vi "barcode main.vi"(8 "error in":errorcluster, 10 "bc station config":T1 {"LIN INFO"."NAD" format="%.0x"; "LIN INFO"."ADCS LIN"."HW select" items=["NI-XNET", "NI-CAN"]; "LVDT Status"."LVDT's stored config"."Lower Limit" format="%.2f"; "LVDT Status"."LVDT's stored config"."Upper Limit" format="%.2f"; "PLC Comms"."PLC string write Tags"."error message 9"."DataSocket Reference"."OnStatusUpdated" format="%.0x"; "PLC Comms"."PLC string write Tags"."error message 9"."DataSocket Reference"."OnDataUpdated" format="%.0x"; "PLC Comms"."PLC string write Tags"."error message 8"."DataSocket Reference"."OnStatusUpdated" format="%.0x"; "PLC Comms"."PLC string write Tags"."error message 8"."DataSocket Reference"."OnDataUpdated" format="%.0x"; "PLC Comms"."PLC string write Tags"."error message 7"."DataSocket Reference"."OnStatusUpdated" format="%.0x"; "PLC Comms"."PLC string write Tags"."error message 7"."DataSocket Reference"."OnDataUpdated" format="%.0x"; "PLC Comms"."PLC string write Tags"."error message 6"."DataSocket Reference"."OnStatusUpdated" format="%.0x"; "PLC Comms"."PLC string write Tags"."error message 6"."DataSocket Reference"."OnDataUpdated" format="%.0x"; "PLC Comms"."PLC string write Tags"."error message 5"."DataSocket Reference"."OnStatusUpdated" format="%.0x"; "PLC Comms"."PLC string write Tags"."error message 5"."DataSocket Reference"."OnDataUpdated" format="%.0x"; "PLC Comms"."PLC string write Tags"."error message 4"."DataSocket Reference"."OnStatusUpdated" format="%.0x"; "PLC Comms"."PLC string write Tags"."error message 4"."DataSocket Reference"."OnDataUpdated" format="%.0x"; "PLC Comms"."PLC string write Tags"."error message 3"."DataSocket Reference"."OnStatusUpdated" format="%.0x"; "PLC Comms"."PLC string write Tags"."error message 3"."DataSocket Reference"."OnDataUpdated" format="%.0x"; "PLC Comms"."PLC string write Tags"."error message 2"."DataSocket Reference"."OnStatusUpdated" format="%.0x"; "PLC Comms"."PLC string write Tags"."error message 2"."DataSocket Reference"."OnDataUpdated" format="%.0x"; "PLC Comms"."PLC string write Tags"."error message 1"."DataSocket Reference"."OnStatusUpdated" format="%.0x"; "PLC Comms"."PLC string write Tags"."error message 1"."DataSocket Reference"."OnDataUpdated" format="%.0x"; "PLC Comms"."PLC string write Tags"."error message 0"."DataSocket Reference"."OnStatusUpdated" format="%.0x"; "PLC Comms"."PLC string write Tags"."error message 0"."DataSocket Reference"."OnDataUpdated" format="%.0x"; "PLC Comms"."PLC string write Tags"."barcode station error"."DataSocket Reference"."OnStatusUpdated" format="%.0x"; "PLC Comms"."PLC string write Tags"."barcode station error"."DataSocket Reference"."OnDataUpdated" format="%.0x"; "PLC Comms"."PLC string read Tags"."iGPS SN 9"."DataSocket Reference"."OnStatusUpdated" format="%.0x"; "PLC Comms"."PLC string read Tags"."iGPS SN 9"."DataSocket Reference"."OnDataUpdated" format="%.0x"; "PLC Comms"."PLC string read Tags"."iGPS SN 8"."DataSocket Reference"."OnStatusUpdated" format="%.0x"; "PLC Comms"."PLC string read Tags"."iGPS SN 8"."DataSocket Reference"."OnDataUpdated" format="%.0x"; "PLC Comms"."PLC string read Tags"."iGPS SN 7"."DataSocket Reference"."OnStatusUpdated" format="%.0x"; "PLC Comms"."PLC string read Tags"."iGPS SN 7"."DataSocket Reference"."OnDataUpdated" format="%.0x"; "PLC Comms"."PLC string read Tags"."iGPS SN 6"."DataSocket Reference"."OnStatusUpdated" format="%.0x"; "PLC Comms"."PLC string read Tags"."iGPS SN 6"."DataSocket Reference"."OnDataUpdated" format="%.0x"; "PLC Comms"."PLC string read Tags"."iGPS SN 5"."DataSocket Reference"."OnStatusUpdated" format="%.0x"; "PLC Comms"."PLC string read Tags"."iGPS SN 5"."DataSocket Reference"."OnDataUpdated" format="%.0x"; "PLC Comms"."PLC string read Tags"."iGPS SN 4"."DataSocket Reference"."OnStatusUpdated" format="%.0x"; "PLC Comms"."PLC string read Tags"."iGPS SN 4"."DataSocket Reference"."OnDataUpdated" format="%.0x"; "PLC Comms"."PLC string read Tags"."iGPS SN 3"."DataSocket Reference"."OnStatusUpdated" format="%.0x"; "PLC Comms"."PLC string read Tags"."iGPS SN 3"."DataSocket Reference"."OnDataUpdated" format="%.0x"; "PLC Comms"."PLC string read Tags"."iGPS SN 2"."DataSocket Reference"."OnStatusUpdated" format="%.0x"; "PLC Comms"."PLC string read Tags"."iGPS SN 2"."DataSocket Reference"."OnDataUpdated" format="%.0x"; "PLC Comms"."PLC string read Tags"."iGPS SN 1"."DataSocket Reference"."OnStatusUpdated" format="%.0x"; "PLC Comms"."PLC string read Tags"."iGPS SN 1"."DataSocket Reference"."OnDataUpdated" format="%.0x"; "PLC Comms"."PLC string read Tags"."iGPS SN 0"."DataSocket Reference"."OnStatusUpdated" format="%.0x"; "PLC Comms"."PLC string read Tags"."iGPS SN 0"."DataSocket Reference"."OnDataUpdated" format="%.0x"; "PLC Comms"."PLC string read Tags"."Manual Part History Number"."DataSocket Reference"."OnStatusUpdated" format="%.0x"; "PLC Comms"."PLC string read Tags"."Manual Part History Number"."DataSocket Reference"."OnDataUpdated" format="%.0x"; "PLC Comms"."PLC string read Tags"."Manual Customer Number"."DataSocket Reference"."OnStatusUpdated" format="%.0x"; "PLC Comms"."PLC string read Tags"."Manual Customer Number"."DataSocket Reference"."OnDataUpdated" format="%.0x"; "PLC Comms"."PLC string read Tags"."Manual Model Type"."DataSocket Reference"."OnStatusUpdated" format="%.0x"; "PLC Comms"."PLC string read Tags"."Manual Model Type"."DataSocket Reference"."OnDataUpdated" format="%.0x"; "PLC Comms"."PLC string read Tags"."Manual Shade Color"."DataSocket Reference"."OnStatusUpdated" format="%.0x"; "PLC Comms"."PLC string read Tags"."Manual Shade Color"."DataSocket Reference"."OnDataUpdated" format="%.0x"; "PLC Comms"."PLC string read Tags"."Manual Inalfa Part Number"."DataSocket Reference"."OnStatusUpdated" format="%.0x"; "PLC Comms"."PLC string read Tags"."Manual Inalfa Part Number"."DataSocket Reference"."OnDataUpdated" format="%.0x"; "PLC Comms"."PLC string read Tags"."Manual Serial Number"."DataSocket Reference"."OnStatusUpdated" format="%.0x"; "PLC Comms"."PLC string read Tags"."Manual Serial Number"."DataSocket Reference"."OnDataUpdated" format="%.0x"; "PLC Comms"."PLC string read Tags"."Shade 2 Barcode"."DataSocket Reference"."OnStatusUpdated" format="%.0x"; "PLC Comms"."PLC string read Tags"."Shade 2 Barcode"."DataSocket Reference"."OnDataUpdated" format="%.0x"; "PLC Comms"."PLC string read Tags"."Shade 1 Barcode"."DataSocket Reference"."OnStatusUpdated" format="%.0x"; "PLC Comms"."PLC string read Tags"."Shade 1 Barcode"."DataSocket Reference"."OnDataUpdated" format="%.0x"; "PLC Comms"."PLC string read Tags"."Part History Number"."DataSocket Reference"."OnStatusUpdated" format="%.0x"; "PLC Comms"."PLC string read Tags"."Part History Number"."DataSocket Reference"."OnDataUpdated" format="%.0x"; "PLC Comms"."PLC string read Tags"."Customer Number"."DataSocket Reference"."OnStatusUpdated" format="%.0x"; "PLC Comms"."PLC string read Tags"."Customer Number"."DataSocket Reference"."OnDataUpdated" format="%.0x"; "PLC Comms"."PLC string read Tags"."Model Type"."DataSocket Reference"."OnStatusUpdated" format="%.0x"; "PLC Comms"."PLC string read Tags"."Model Type"."DataSocket Reference"."OnDataUpdated" format="%.0x"; "PLC Comms"."PLC string read Tags"."Shade Color"."DataSocket Reference"."OnStatusUpdated" format="%.0x"; "PLC Comms"."PLC string read Tags"."Shade Color"."DataSocket Reference"."OnDataUpdated" format="%.0x"; "PLC Comms"."PLC string read Tags"."Inalfa Part Number"."DataSocket Reference"."OnStatusUpdated" format="%.0x"; "PLC Comms"."PLC string read Tags"."Inalfa Part Number"."DataSocket Reference"."OnDataUpdated" format="%.0x"; "PLC Comms"."PLC string read Tags"."Pallet Number"."DataSocket Reference"."OnStatusUpdated" format="%.0x"; "PLC Comms"."PLC string read Tags"."Pallet Number"."DataSocket Reference"."OnDataUpdated" format="%.0x"; "PLC Comms"."PLC string read Tags"."Serial Number"."DataSocket Reference"."OnStatusUpdated" format="%.0x"; "PLC Comms"."PLC string read Tags"."Serial Number"."DataSocket Reference"."OnDataUpdated" format="%.0x"; "PLC Comms"."PLC bool write Tags"."Move LVDT Adjust Station"."DataSocket Reference"."OnStatusUpdated" format="%.0x"; "PLC Comms"."PLC bool write Tags"."Move LVDT Adjust Station"."DataSocket Reference"."OnDataUpdated" format="%.0x"; "PLC Comms"."PLC bool write Tags"."AT set to Vent ATS Home Pos"."DataSocket Reference"."OnStatusUpdated" format="%.0x"; "PLC Comms"."PLC bool write Tags"."AT set to Vent ATS Home Pos"."DataSocket Reference"."OnDataUpdated" format="%.0x"; "PLC Comms"."PLC bool write Tags"."AT set to Vent ATS Test Pos"."DataSocket Reference"."OnStatusUpdated" format="%.0x"; "PLC Comms"."PLC bool write Tags"."AT set to Vent ATS Test Pos"."DataSocket Reference"."OnDataUpdated" format="%.0x"; "PLC Comms"."PLC bool write Tags"."Barcode02 OK"."DataSocket Reference"."OnStatusUpdated" format="%.0x"; "PLC Comms"."PLC bool write Tags"."Barcode02 OK"."DataSocket Reference"."OnDataUpdated" format="%.0x"; "PLC Comms"."PLC bool write Tags"."Barcode01 OK"."DataSocket Reference"."OnStatusUpdated" format="%.0x"; "PLC Comms"."PLC bool write Tags"."Barcode01 OK"."DataSocket Reference"."OnDataUpdated" format="%.0x"; "PLC Comms"."PLC bool write Tags"."AT set wand 02 home pos"."DataSocket Reference"."OnStatusUpdated" format="%.0x"; "PLC Comms"."PLC bool write Tags"."AT set wand 02 home pos"."DataSocket Reference"."OnDataUpdated" format="%.0x"; "PLC Comms"."PLC bool write Tags"."AT set sunshade 02 wand up"."DataSocket Reference"."OnStatusUpdated" format="%.0x"; "PLC Comms"."PLC bool write Tags"."AT set sunshade 02 wand up"."DataSocket Reference"."OnDataUpdated" format="%.0x"; "PLC Comms"."PLC bool write Tags"."NVH Operator Finish"."DataSocket Reference"."OnStatusUpdated" format="%.0x"; "PLC Comms"."PLC bool write Tags"."NVH Operator Finish"."DataSocket Reference"."OnDataUpdated" format="%.0x"; "PLC Comms"."PLC bool write Tags"."NVH Operator Glass Close Noise"."DataSocket Reference"."OnStatusUpdated" format="%.0x"; "PLC Comms"."PLC bool write Tags"."NVH Operator Glass Close Noise"."DataSocket Reference"."OnDataUpdated" format="%.0x"; "PLC Comms"."PLC bool write Tags"."NVH Operator Glass Open Noise"."DataSocket Reference"."OnStatusUpdated" format="%.0x"; "PLC Comms"."PLC bool write Tags"."NVH Operator Glass Open Noise"."DataSocket Reference"."OnDataUpdated" format="%.0x"; "PLC Comms"."PLC bool write Tags"."NVH Operator Sunshade Close Noise"."DataSocket Reference"."OnStatusUpdated" format="%.0x"; "PLC Comms"."PLC bool write Tags"."NVH Operator Sunshade Close Noise"."DataSocket Reference"."OnDataUpdated" format="%.0x"; "PLC Comms"."PLC bool write Tags"."NVH Operator Sunshade Open Noise"."DataSocket Reference"."OnStatusUpdated" format="%.0x"; "PLC Comms"."PLC bool write Tags"."NVH Operator Sunshade Open Noise"."DataSocket Reference"."OnDataUpdated" format="%.0x"; "PLC Comms"."PLC bool write Tags"."NVH Operator Vent Close Noise"."DataSocket Reference"."OnStatusUpdated" format="%.0x"; "PLC Comms"."PLC bool write Tags"."NVH Operator Vent Close Noise"."DataSocket Reference"."OnDataUpdated" format="%.0x"; "PLC Comms"."PLC bool write Tags"."NVH Operator Vent Open Noise"."DataSocket Reference"."OnStatusUpdated" format="%.0x"; "PLC Comms"."PLC bool write Tags"."NVH Operator Vent Open Noise"."DataSocket Reference"."OnDataUpdated" format="%.0x"; "PLC Comms"."PLC bool write Tags"."NVH Operator Check"."DataSocket Reference"."OnStatusUpdated" format="%.0x"; "PLC Comms"."PLC bool write Tags"."NVH Operator Check"."DataSocket Reference"."OnDataUpdated" format="%.0x"; "PLC Comms"."PLC bool write Tags"."NVH Operator Fail"."DataSocket Reference"."OnStatusUpdated" format="%.0x"; "PLC Comms"."PLC bool write Tags"."NVH Operator Fail"."DataSocket Reference"."OnDataUpdated" format="%.0x"; "PLC Comms"."PLC bool write Tags"."NVH Operator Pass"."DataSocket Reference"."OnStatusUpdated" format="%.0x"; "PLC Comms"."PLC bool write Tags"."NVH Operator Pass"."DataSocket Reference"."OnDataUpdated" format="%.0x"; "PLC Comms"."PLC bool write Tags"."NVH Operator Express Rollo Opened02"."DataSocket Reference"."OnStatusUpdated" format="%.0x"; "PLC Comms"."PLC bool write Tags"."NVH Operator Express Rollo Opened02"."DataSocket Reference"."OnDataUpdated" format="%.0x"; "PLC Comms"."PLC bool write Tags"."NVH Operator Express Rollo Closed01"."DataSocket Reference"."OnStatusUpdated" format="%.0x"; "PLC Comms"."PLC bool write Tags"."NVH Operator Express Rollo Closed01"."DataSocket Reference"."OnDataUpdated" format="%.0x"; "PLC Comms"."PLC bool write Tags"."NVH Operator Express Rollo Opened01"."DataSocket Reference"."OnStatusUpdated" format="%.0x"; "PLC Comms"."PLC bool write Tags"."NVH Operator Express Rollo Opened01"."DataSocket Reference"."OnDataUpdated" format="%.0x"; "PLC Comms"."PLC bool write Tags"."NVH Operator Express Glass Closed"."DataSocket Reference"."OnStatusUpdated" format="%.0x"; "PLC Comms"."PLC bool write Tags"."NVH Operator Express Glass Closed"."DataSocket Reference"."OnDataUpdated" format="%.0x"; "PLC Comms"."PLC bool write Tags"."NVH Operator Express Glass Opened"."DataSocket Reference"."OnStatusUpdated" format="%.0x"; "PLC Comms"."PLC bool write Tags"."NVH Operator Express Glass Opened"."DataSocket Reference"."OnDataUpdated" format="%.0x"; "PLC Comms"."PLC bool write Tags"."NVH Fail"."DataSocket Reference"."OnStatusUpdated" format="%.0x"; "PLC Comms"."PLC bool write Tags"."NVH Fail"."DataSocket Reference"."OnDataUpdated" format="%.0x"; "PLC Comms"."PLC bool write Tags"."NVH Pass"."DataSocket Reference"."OnStatusUpdated" format="%.0x"; "PLC Comms"."PLC bool write Tags"."NVH Pass"."DataSocket Reference"."OnDataUpdated" format="%.0x"; "PLC Comms"."PLC bool write Tags"."NVH SunRoof Stop"."DataSocket Reference"."OnStatusUpdated" format="%.0x"; "PLC Comms"."PLC bool write Tags"."NVH SunRoof Stop"."DataSocket Reference"."OnDataUpdated" format="%.0x"; "PLC Comms"."PLC bool write Tags"."NVH SunRoof Moving"."DataSocket Reference"."OnStatusUpdated" format="%.0x"; "PLC Comms"."PLC bool write Tags"."NVH SunRoof Moving"."DataSocket Reference"."OnDataUpdated" format="%.0x"; "PLC Comms"."PLC bool write Tags"."Extend Z LVDTS"."DataSocket Reference"."OnStatusUpdated" format="%.0x"; "PLC Comms"."PLC bool write Tags"."Extend Z LVDTS"."DataSocket Reference"."OnDataUpdated" format="%.0x"; "PLC Comms"."PLC bool write Tags"."Bad Frame Barcode"."DataSocket Reference"."OnStatusUpdated" format="%.0x"; "PLC Comms"."PLC bool write Tags"."Bad Frame Barcode"."DataSocket Reference"."OnDataUpdated" format="%.0x"; "PLC Comms"."PLC bool write Tags"."Good Frame Barcode"."DataSocket Reference"."OnStatusUpdated" format="%.0x"; "PLC Comms"."PLC bool write Tags"."Good Frame Barcode"."DataSocket Reference"."OnDataUpdated" format="%.0x"; "PLC Comms"."PLC bool write Tags"."AT VentPMACExtended"."DataSocket Reference"."OnStatusUpdated" format="%.0x"; "PLC Comms"."PLC bool write Tags"."AT VentPMACExtended"."DataSocket Reference"."OnDataUpdated" format="%.0x"; "PLC Comms"."PLC bool write Tags"."AT VentPMACHome"."DataSocket Reference"."OnStatusUpdated" format="%.0x"; "PLC Comms"."PLC bool write Tags"."AT VentPMACHome"."DataSocket Reference"."OnDataUpdated" format="%.0x"; "PLC Comms"."PLC bool write Tags"."control slide stop"."DataSocket Reference"."OnStatusUpdated" format="%.0x"; "PLC Comms"."PLC bool write Tags"."control slide stop"."DataSocket Reference"."OnDataUpdated" format="%.0x"; "PLC Comms"."PLC bool write Tags"."control slide start"."DataSocket Reference"."OnStatusUpdated" format="%.0x"; "PLC Comms"."PLC bool write Tags"."control slide start"."DataSocket Reference"."OnDataUpdated" format="%.0x"; "PLC Comms"."PLC bool write Tags"."ss servo close"."DataSocket Reference"."OnStatusUpdated" format="%.0x"; "PLC Comms"."PLC bool write Tags"."ss servo close"."DataSocket Reference"."OnDataUpdated" format="%.0x"; "PLC Comms"."PLC bool write Tags"."ss servo open"."DataSocket Reference"."OnStatusUpdated" format="%.0x"; "PLC Comms"."PLC bool write Tags"."ss servo open"."DataSocket Reference"."OnDataUpdated" format="%.0x"; "PLC Comms"."PLC bool write Tags"."Extend LVDT's"."DataSocket Reference"."OnStatusUpdated" format="%.0x"; "PLC Comms"."PLC bool write Tags"."Extend LVDT's"."DataSocket Reference"."OnDataUpdated" format="%.0x"; "PLC Comms"."PLC bool write Tags"."Retract LVDT's"."DataSocket Reference"."OnStatusUpdated" format="%.0x"; "PLC Comms"."PLC bool write Tags"."Retract LVDT's"."DataSocket Reference"."OnDataUpdated" format="%.0x"; "PLC Comms"."PLC bool write Tags"."Test Started"."DataSocket Reference"."OnStatusUpdated" format="%.0x"; "PLC Comms"."PLC bool write Tags"."Test Started"."DataSocket Reference"."OnDataUpdated" format="%.0x"; "PLC Comms"."PLC bool write Tags"."Test Complete Fail"."DataSocket Reference"."OnStatusUpdated" format="%.0x"; "PLC Comms"."PLC bool write Tags"."Test Complete Fail"."DataSocket Reference"."OnDataUpdated" format="%.0x"; "PLC Comms"."PLC bool write Tags"."Test Complete Pass"."DataSocket Reference"."OnStatusUpdated" format="%.0x"; "PLC Comms"."PLC bool write Tags"."Test Complete Pass"."DataSocket Reference"."OnDataUpdated" format="%.0x"; "PLC Comms"."PLC bool write Tags"."AT set wand home pos"."DataSocket Reference"."OnStatusUpdated" format="%.0x"; "PLC Comms"."PLC bool write Tags"."AT set wand home pos"."DataSocket Reference"."OnDataUpdated" format="%.0x"; "PLC Comms"."PLC bool write Tags"."AT set sunshade wand lower"."DataSocket Reference"."OnStatusUpdated" format="%.0x"; "PLC Comms"."PLC bool write Tags"."AT set sunshade wand lower"."DataSocket Reference"."OnDataUpdated" format="%.0x"; "PLC Comms"."PLC bool write Tags"."AT set glass wand lower"."DataSocket Reference"."OnStatusUpdated" format="%.0x"; "PLC Comms"."PLC bool write Tags"."AT set glass wand lower"."DataSocket Reference"."OnDataUpdated" format="%.0x"; "PLC Comms"."PLC boolean read Tags"."Finish Adjust LVDT"."DataSocket Reference"."OnStatusUpdated" format="%.0x"; "PLC Comms"."PLC boolean read Tags"."Finish Adjust LVDT"."DataSocket Reference"."OnDataUpdated" format="%.0x"; "PLC Comms"."PLC boolean read Tags"."Start Adjust LVDT"."DataSocket Reference"."OnStatusUpdated" format="%.0x"; "PLC Comms"."PLC boolean read Tags"."Start Adjust LVDT"."DataSocket Reference"."OnDataUpdated" format="%.0x"; "PLC Comms"."PLC boolean read Tags"."AT at vent ATS Home pos"."DataSocket Reference"."OnStatusUpdated" format="%.0x"; "PLC Comms"."PLC boolean read Tags"."AT at vent ATS Home pos"."DataSocket Reference"."OnDataUpdated" format="%.0x"; "PLC Comms"."PLC boolean read Tags"."AT at vent ATS test pos"."DataSocket Reference"."OnStatusUpdated" format="%.0x"; "PLC Comms"."PLC boolean read Tags"."AT at vent ATS test pos"."DataSocket Reference"."OnDataUpdated" format="%.0x"; "PLC Comms"."PLC boolean read Tags"."NVH Operator Re-do"."DataSocket Reference"."OnStatusUpdated" format="%.0x"; "PLC Comms"."PLC boolean read Tags"."NVH Operator Re-do"."DataSocket Reference"."OnDataUpdated" format="%.0x"; "PLC Comms"."PLC boolean read Tags"."NVH Operator Express Glass Vent Close"."DataSocket Reference"."OnStatusUpdated" format="%.0x"; "PLC Comms"."PLC boolean read Tags"."NVH Operator Express Glass Vent Close"."DataSocket Reference"."OnDataUpdated" format="%.0x"; "PLC Comms"."PLC boolean read Tags"."NVH Operator Express Glass vent Open"."DataSocket Reference"."OnStatusUpdated" format="%.0x"; "PLC Comms"."PLC boolean read Tags"."NVH Operator Express Glass vent Open"."DataSocket Reference"."OnDataUpdated" format="%.0x"; "PLC Comms"."PLC boolean read Tags"."windproof position"."DataSocket Reference"."OnStatusUpdated" format="%.0x"; "PLC Comms"."PLC boolean read Tags"."windproof position"."DataSocket Reference"."OnDataUpdated" format="%.0x"; "PLC Comms"."PLC boolean read Tags"."AT in wand 02 home pos"."DataSocket Reference"."OnStatusUpdated" format="%.0x"; "PLC Comms"."PLC boolean read Tags"."AT in wand 02 home pos"."DataSocket Reference"."OnDataUpdated" format="%.0x"; "PLC Comms"."PLC boolean read Tags"."AT in sunshad 02 wand up pos"."DataSocket Reference"."OnStatusUpdated" format="%.0x"; "PLC Comms"."PLC boolean read Tags"."AT in sunshad 02 wand up pos"."DataSocket Reference"."OnDataUpdated" format="%.0x"; "PLC Comms"."PLC boolean read Tags"."AT shade 02 position"."DataSocket Reference"."OnStatusUpdated" format="%.0x"; "PLC Comms"."PLC boolean read Tags"."AT shade 02 position"."DataSocket Reference"."OnDataUpdated" format="%.0x"; "PLC Comms"."PLC boolean read Tags"."NVH Operator Check"."DataSocket Reference"."OnStatusUpdated" format="%.0x"; "PLC Comms"."PLC boolean read Tags"."NVH Operator Check"."DataSocket Reference"."OnDataUpdated" format="%.0x"; "PLC Comms"."PLC boolean read Tags"."NVH Operator Finish"."DataSocket Reference"."OnStatusUpdated" format="%.0x"; "PLC Comms"."PLC boolean read Tags"."NVH Operator Finish"."DataSocket Reference"."OnDataUpdated" format="%.0x"; "PLC Comms"."PLC boolean read Tags"."NVH Operator Glass Close Noise"."DataSocket Reference"."OnStatusUpdated" format="%.0x"; "PLC Comms"."PLC boolean read Tags"."NVH Operator Glass Close Noise"."DataSocket Reference"."OnDataUpdated" format="%.0x"; "PLC Comms"."PLC boolean read Tags"."NVH Operator Glass Open Noise"."DataSocket Reference"."OnStatusUpdated" format="%.0x"; "PLC Comms"."PLC boolean read Tags"."NVH Operator Glass Open Noise"."DataSocket Reference"."OnDataUpdated" format="%.0x"; "PLC Comms"."PLC boolean read Tags"."NVH Operator Sunshade Close Noise"."DataSocket Reference"."OnStatusUpdated" format="%.0x"; "PLC Comms"."PLC boolean read Tags"."NVH Operator Sunshade Close Noise"."DataSocket Reference"."OnDataUpdated" format="%.0x"; "PLC Comms"."PLC boolean read Tags"."NVH Operator Sunshade Open Noise"."DataSocket Reference"."OnStatusUpdated" format="%.0x"; "PLC Comms"."PLC boolean read Tags"."NVH Operator Sunshade Open Noise"."DataSocket Reference"."OnDataUpdated" format="%.0x"; "PLC Comms"."PLC boolean read Tags"."NVH Operator Vent Close Noise"."DataSocket Reference"."OnStatusUpdated" format="%.0x"; "PLC Comms"."PLC boolean read Tags"."NVH Operator Vent Close Noise"."DataSocket Reference"."OnDataUpdated" format="%.0x"; "PLC Comms"."PLC boolean read Tags"."NVH Operator Vent Open Noise"."DataSocket Reference"."OnStatusUpdated" format="%.0x"; "PLC Comms"."PLC boolean read Tags"."NVH Operator Vent Open Noise"."DataSocket Reference"."OnDataUpdated" format="%.0x"; "PLC Comms"."PLC boolean read Tags"."NVH Operator Express Rollo Close02"."DataSocket Reference"."OnStatusUpdated" format="%.0x"; "PLC Comms"."PLC boolean read Tags"."NVH Operator Express Rollo Close02"."DataSocket Reference"."OnDataUpdated" format="%.0x"; "PLC Comms"."PLC boolean read Tags"."NVH Operator Express Rollo Open02"."DataSocket Reference"."OnStatusUpdated" format="%.0x"; "PLC Comms"."PLC boolean read Tags"."NVH Operator Express Rollo Open02"."DataSocket Reference"."OnDataUpdated" format="%.0x"; "PLC Comms"."PLC boolean read Tags"."NVH Operator Express Rollo Close01"."DataSocket Reference"."OnStatusUpdated" format="%.0x"; "PLC Comms"."PLC boolean read Tags"."NVH Operator Express Rollo Close01"."DataSocket Reference"."OnDataUpdated" format="%.0x"; "PLC Comms"."PLC boolean read Tags"."NVH Operator Express Rollo Open01"."DataSocket Reference"."OnStatusUpdated" format="%.0x"; "PLC Comms"."PLC boolean read Tags"."NVH Operator Express Rollo Open01"."DataSocket Reference"."OnDataUpdated" format="%.0x"; "PLC Comms"."PLC boolean read Tags"."NVH Operator Express Glass Close"."DataSocket Reference"."OnStatusUpdated" format="%.0x"; "PLC Comms"."PLC boolean read Tags"."NVH Operator Express Glass Close"."DataSocket Reference"."OnDataUpdated" format="%.0x"; "PLC Comms"."PLC boolean read Tags"."NVH Operator Express Glass Open"."DataSocket Reference"."OnStatusUpdated" format="%.0x"; "PLC Comms"."PLC boolean read Tags"."NVH Operator Express Glass Open"."DataSocket Reference"."OnDataUpdated" format="%.0x"; "PLC Comms"."PLC boolean read Tags"."NVH Operator Fail"."DataSocket Reference"."OnStatusUpdated" format="%.0x"; "PLC Comms"."PLC boolean read Tags"."NVH Operator Fail"."DataSocket Reference"."OnDataUpdated" format="%.0x"; "PLC Comms"."PLC boolean read Tags"."NVH Operator Pass"."DataSocket Reference"."OnStatusUpdated" format="%.0x"; "PLC Comms"."PLC boolean read Tags"."NVH Operator Pass"."DataSocket Reference"."OnDataUpdated" format="%.0x"; "PLC Comms"."PLC boolean read Tags"."Z LVDTs Extended"."DataSocket Reference"."OnStatusUpdated" format="%.0x"; "PLC Comms"."PLC boolean read Tags"."Z LVDTs Extended"."DataSocket Reference"."OnDataUpdated" format="%.0x"; "PLC Comms"."PLC boolean read Tags"."iGPS Pass 9"."DataSocket Reference"."OnStatusUpdated" format="%.0x"; "PLC Comms"."PLC boolean read Tags"."iGPS Pass 9"."DataSocket Reference"."OnDataUpdated" format="%.0x"; "PLC Comms"."PLC boolean read Tags"."iGPS Pass 8"."DataSocket Reference"."OnStatusUpdated" format="%.0x"; "PLC Comms"."PLC boolean read Tags"."iGPS Pass 8"."DataSocket Reference"."OnDataUpdated" format="%.0x"; "PLC Comms"."PLC boolean read Tags"."iGPS Pass 7"."DataSocket Reference"."OnStatusUpdated" format="%.0x"; "PLC Comms"."PLC boolean read Tags"."iGPS Pass 7"."DataSocket Reference"."OnDataUpdated" format="%.0x"; "PLC Comms"."PLC boolean read Tags"."iGPS Pass 6"."DataSocket Reference"."OnStatusUpdated" format="%.0x"; "PLC Comms"."PLC boolean read Tags"."iGPS Pass 6"."DataSocket Reference"."OnDataUpdated" format="%.0x"; "PLC Comms"."PLC boolean read Tags"."iGPS Pass 5"."DataSocket Reference"."OnStatusUpdated" format="%.0x"; "PLC Comms"."PLC boolean read Tags"."iGPS Pass 5"."DataSocket Reference"."OnDataUpdated" format="%.0x"; "PLC Comms"."PLC boolean read Tags"."iGPS Pass 4"."DataSocket Reference"."OnStatusUpdated" format="%.0x"; "PLC Comms"."PLC boolean read Tags"."iGPS Pass 4"."DataSocket Reference"."OnDataUpdated" format="%.0x"; "PLC Comms"."PLC boolean read Tags"."iGPS Pass 3"."DataSocket Reference"."OnStatusUpdated" format="%.0x"; "PLC Comms"."PLC boolean read Tags"."iGPS Pass 3"."DataSocket Reference"."OnDataUpdated" format="%.0x"; "PLC Comms"."PLC boolean read Tags"."iGPS Pass 2"."DataSocket Reference"."OnStatusUpdated" format="%.0x"; "PLC Comms"."PLC boolean read Tags"."iGPS Pass 2"."DataSocket Reference"."OnDataUpdated" format="%.0x"; "PLC Comms"."PLC boolean read Tags"."iGPS Pass 1"."DataSocket Reference"."OnStatusUpdated" format="%.0x"; "PLC Comms"."PLC boolean read Tags"."iGPS Pass 1"."DataSocket Reference"."OnDataUpdated" format="%.0x"; "PLC Comms"."PLC boolean read Tags"."iGPS Pass 0"."DataSocket Reference"."OnStatusUpdated" format="%.0x"; "PLC Comms"."PLC boolean read Tags"."iGPS Pass 0"."DataSocket Reference"."OnDataUpdated" format="%.0x"; "PLC Comms"."PLC boolean read Tags"."Check Frame Barcode"."DataSocket Reference"."OnStatusUpdated" format="%.0x"; "PLC Comms"."PLC boolean read Tags"."Check Frame Barcode"."DataSocket Reference"."OnDataUpdated" format="%.0x"; "PLC Comms"."PLC boolean read Tags"."SS Barcode Scanner Bypassed"."DataSocket Reference"."OnStatusUpdated" format="%.0x"; "PLC Comms"."PLC boolean read Tags"."SS Barcode Scanner Bypassed"."DataSocket Reference"."OnDataUpdated" format="%.0x"; "PLC Comms"."PLC boolean read Tags"."AT VentPMACisExtend"."DataSocket Reference"."OnStatusUpdated" format="%.0x"; "PLC Comms"."PLC boolean read Tags"."AT VentPMACisExtend"."DataSocket Reference"."OnDataUpdated" format="%.0x"; "PLC Comms"."PLC boolean read Tags"."AT VentPMACatHome"."DataSocket Reference"."OnStatusUpdated" format="%.0x"; "PLC Comms"."PLC boolean read Tags"."AT VentPMACatHome"."DataSocket Reference"."OnDataUpdated" format="%.0x"; "PLC Comms"."PLC boolean read Tags"."wind deflector low speed pos"."DataSocket Reference"."OnStatusUpdated" format="%.0x"; "PLC Comms"."PLC boolean read Tags"."wind deflector low speed pos"."DataSocket Reference"."OnDataUpdated" format="%.0x"; "PLC Comms"."PLC boolean read Tags"."wind deflector high speed pos"."DataSocket Reference"."OnStatusUpdated" format="%.0x"; "PLC Comms"."PLC boolean read Tags"."wind deflector high speed pos"."DataSocket Reference"."OnDataUpdated" format="%.0x"; "PLC Comms"."PLC boolean read Tags"."control slide right over stroke"."DataSocket Reference"."OnStatusUpdated" format="%.0x"; "PLC Comms"."PLC boolean read Tags"."control slide right over stroke"."DataSocket Reference"."OnDataUpdated" format="%.0x"; "PLC Comms"."PLC boolean read Tags"."control slide right good"."DataSocket Reference"."OnStatusUpdated" format="%.0x"; "PLC Comms"."PLC boolean read Tags"."control slide right good"."DataSocket Reference"."OnDataUpdated" format="%.0x"; "PLC Comms"."PLC boolean read Tags"."control slide left over stroke"."DataSocket Reference"."OnStatusUpdated" format="%.0x"; "PLC Comms"."PLC boolean read Tags"."control slide left over stroke"."DataSocket Reference"."OnDataUpdated" format="%.0x"; "PLC Comms"."PLC boolean read Tags"."control slide left good"."DataSocket Reference"."OnStatusUpdated" format="%.0x"; "PLC Comms"."PLC boolean read Tags"."control slide left good"."DataSocket Reference"."OnDataUpdated" format="%.0x"; "PLC Comms"."PLC boolean read Tags"."control slide at home"."DataSocket Reference"."OnStatusUpdated" format="%.0x"; "PLC Comms"."PLC boolean read Tags"."control slide at home"."DataSocket Reference"."OnDataUpdated" format="%.0x"; "PLC Comms"."PLC boolean read Tags"."ss servo closing"."DataSocket Reference"."OnStatusUpdated" format="%.0x"; "PLC Comms"."PLC boolean read Tags"."ss servo closing"."DataSocket Reference"."OnDataUpdated" format="%.0x"; "PLC Comms"."PLC boolean read Tags"."ss servo opening"."DataSocket Reference"."OnStatusUpdated" format="%.0x"; "PLC Comms"."PLC boolean read Tags"."ss servo opening"."DataSocket Reference"."OnDataUpdated" format="%.0x"; "PLC Comms"."PLC boolean read Tags"."ss servo at close"."DataSocket Reference"."OnStatusUpdated" format="%.0x"; "PLC Comms"."PLC boolean read Tags"."ss servo at close"."DataSocket Reference"."OnDataUpdated" format="%.0x"; "PLC Comms"."PLC boolean read Tags"."ss servo at open"."DataSocket Reference"."OnStatusUpdated" format="%.0x"; "PLC Comms"."PLC boolean read Tags"."ss servo at open"."DataSocket Reference"."OnDataUpdated" format="%.0x"; "PLC Comms"."PLC boolean read Tags"."manual barcode print"."DataSocket Reference"."OnStatusUpdated" format="%.0x"; "PLC Comms"."PLC boolean read Tags"."manual barcode print"."DataSocket Reference"."OnDataUpdated" format="%.0x"; "PLC Comms"."PLC boolean read Tags"."LVDT's Retracted"."DataSocket Reference"."OnStatusUpdated" format="%.0x"; "PLC Comms"."PLC boolean read Tags"."LVDT's Retracted"."DataSocket Reference"."OnDataUpdated" format="%.0x"; "PLC Comms"."PLC boolean read Tags"."abort"."DataSocket Reference"."OnStatusUpdated" format="%.0x"; "PLC Comms"."PLC boolean read Tags"."abort"."DataSocket Reference"."OnDataUpdated" format="%.0x"; "PLC Comms"."PLC boolean read Tags"."start"."DataSocket Reference"."OnStatusUpdated" format="%.0x"; "PLC Comms"."PLC boolean read Tags"."start"."DataSocket Reference"."OnDataUpdated" format="%.0x"; "PLC Comms"."PLC boolean read Tags"."bolt check 21"."DataSocket Reference"."OnStatusUpdated" format="%.0x"; "PLC Comms"."PLC boolean read Tags"."bolt check 21"."DataSocket Reference"."OnDataUpdated" format="%.0x"; "PLC Comms"."PLC boolean read Tags"."bolt check 20"."DataSocket Reference"."OnStatusUpdated" format="%.0x"; "PLC Comms"."PLC boolean read Tags"."bolt check 20"."DataSocket Reference"."OnDataUpdated" format="%.0x"; "PLC Comms"."PLC boolean read Tags"."bolt check 19"."DataSocket Reference"."OnStatusUpdated" format="%.0x"; "PLC Comms"."PLC boolean read Tags"."bolt check 19"."DataSocket Reference"."OnDataUpdated" format="%.0x"; "PLC Comms"."PLC boolean read Tags"."bolt check 18"."DataSocket Reference"."OnStatusUpdated" format="%.0x"; "PLC Comms"."PLC boolean read Tags"."bolt check 18"."DataSocket Reference"."OnDataUpdated" format="%.0x"; "PLC Comms"."PLC boolean read Tags"."bolt check 17"."DataSocket Reference"."OnStatusUpdated" format="%.0x"; "PLC Comms"."PLC boolean read Tags"."bolt check 17"."DataSocket Reference"."OnDataUpdated" format="%.0x"; "PLC Comms"."PLC boolean read Tags"."bolt check 16"."DataSocket Reference"."OnStatusUpdated" format="%.0x"; "PLC Comms"."PLC boolean read Tags"."bolt check 16"."DataSocket Reference"."OnDataUpdated" format="%.0x"; "PLC Comms"."PLC boolean read Tags"."bolt check 15"."DataSocket Reference"."OnStatusUpdated" format="%.0x"; "PLC Comms"."PLC boolean read Tags"."bolt check 15"."DataSocket Reference"."OnDataUpdated" format="%.0x"; "PLC Comms"."PLC boolean read Tags"."bolt check 14"."DataSocket Reference"."OnStatusUpdated" format="%.0x"; "PLC Comms"."PLC boolean read Tags"."bolt check 14"."DataSocket Reference"."OnDataUpdated" format="%.0x"; "PLC Comms"."PLC boolean read Tags"."bolt check 13"."DataSocket Reference"."OnStatusUpdated" format="%.0x"; "PLC Comms"."PLC boolean read Tags"."bolt check 13"."DataSocket Reference"."OnDataUpdated" format="%.0x"; "PLC Comms"."PLC boolean read Tags"."bolt check 12"."DataSocket Reference"."OnStatusUpdated" format="%.0x"; "PLC Comms"."PLC boolean read Tags"."bolt check 12"."DataSocket Reference"."OnDataUpdated" format="%.0x"; "PLC Comms"."PLC boolean read Tags"."bolt check 11"."DataSocket Reference"."OnStatusUpdated" format="%.0x"; "PLC Comms"."PLC boolean read Tags"."bolt check 11"."DataSocket Reference"."OnDataUpdated" format="%.0x"; "PLC Comms"."PLC boolean read Tags"."bolt check 10"."DataSocket Reference"."OnStatusUpdated" format="%.0x"; "PLC Comms"."PLC boolean read Tags"."bolt check 10"."DataSocket Reference"."OnDataUpdated" format="%.0x"; "PLC Comms"."PLC boolean read Tags"."bolt check 9"."DataSocket Reference"."OnStatusUpdated" format="%.0x"; "PLC Comms"."PLC boolean read Tags"."bolt check 9"."DataSocket Reference"."OnDataUpdated" format="%.0x"; "PLC Comms"."PLC boolean read Tags"."bolt check 8"."DataSocket Reference"."OnStatusUpdated" format="%.0x"; "PLC Comms"."PLC boolean read Tags"."bolt check 8"."DataSocket Reference"."OnDataUpdated" format="%.0x"; "PLC Comms"."PLC boolean read Tags"."bolt check 7"."DataSocket Reference"."OnStatusUpdated" format="%.0x"; "PLC Comms"."PLC boolean read Tags"."bolt check 7"."DataSocket Reference"."OnDataUpdated" format="%.0x"; "PLC Comms"."PLC boolean read Tags"."bolt check 6"."DataSocket Reference"."OnStatusUpdated" format="%.0x"; "PLC Comms"."PLC boolean read Tags"."bolt check 6"."DataSocket Reference"."OnDataUpdated" format="%.0x"; "PLC Comms"."PLC boolean read Tags"."bolt check 5"."DataSocket Reference"."OnStatusUpdated" format="%.0x"; "PLC Comms"."PLC boolean read Tags"."bolt check 5"."DataSocket Reference"."OnDataUpdated" format="%.0x"; "PLC Comms"."PLC boolean read Tags"."bolt check 4"."DataSocket Reference"."OnStatusUpdated" format="%.0x"; "PLC Comms"."PLC boolean read Tags"."bolt check 4"."DataSocket Reference"."OnDataUpdated" format="%.0x"; "PLC Comms"."PLC boolean read Tags"."bolt check 3"."DataSocket Reference"."OnStatusUpdated" format="%.0x"; "PLC Comms"."PLC boolean read Tags"."bolt check 3"."DataSocket Reference"."OnDataUpdated" format="%.0x"; "PLC Comms"."PLC boolean read Tags"."bolt check 2"."DataSocket Reference"."OnStatusUpdated" format="%.0x"; "PLC Comms"."PLC boolean read Tags"."bolt check 2"."DataSocket Reference"."OnDataUpdated" format="%.0x"; "PLC Comms"."PLC boolean read Tags"."bolt check 1"."DataSocket Reference"."OnStatusUpdated" format="%.0x"; "PLC Comms"."PLC boolean read Tags"."bolt check 1"."DataSocket Reference"."OnDataUpdated" format="%.0x"; "PLC Comms"."PLC boolean read Tags"."FB light block present"."DataSocket Reference"."OnStatusUpdated" format="%.0x"; "PLC Comms"."PLC boolean read Tags"."FB light block present"."DataSocket Reference"."OnDataUpdated" format="%.0x"; "PLC Comms"."PLC boolean read Tags"."audit gap hider present RH"."DataSocket Reference"."OnStatusUpdated" format="%.0x"; "PLC Comms"."PLC boolean read Tags"."audit gap hider present RH"."DataSocket Reference"."OnDataUpdated" format="%.0x"; "PLC Comms"."PLC boolean read Tags"."audit gap hider present LH"."DataSocket Reference"."OnStatusUpdated" format="%.0x"; "PLC Comms"."PLC boolean read Tags"."audit gap hider present LH"."DataSocket Reference"."OnDataUpdated" format="%.0x"; "PLC Comms"."PLC boolean read Tags"."motor foam present RH"."DataSocket Reference"."OnStatusUpdated" format="%.0x"; "PLC Comms"."PLC boolean read Tags"."motor foam present RH"."DataSocket Reference"."OnDataUpdated" format="%.0x"; "PLC Comms"."PLC boolean read Tags"."motor foam present LH"."DataSocket Reference"."OnStatusUpdated" format="%.0x"; "PLC Comms"."PLC boolean read Tags"."motor foam present LH"."DataSocket Reference"."OnDataUpdated" format="%.0x"; "PLC Comms"."PLC boolean read Tags"."LVDT's Extended"."DataSocket Reference"."OnStatusUpdated" format="%.0x"; "PLC Comms"."PLC boolean read Tags"."LVDT's Extended"."DataSocket Reference"."OnDataUpdated" format="%.0x"; "PLC Comms"."PLC boolean read Tags"."AT in wand home pos"."DataSocket Reference"."OnStatusUpdated" format="%.0x"; "PLC Comms"."PLC boolean read Tags"."AT in wand home pos"."DataSocket Reference"."OnDataUpdated" format="%.0x"; "PLC Comms"."PLC boolean read Tags"."AT in sunshad wand lower pos"."DataSocket Reference"."OnStatusUpdated" format="%.0x"; "PLC Comms"."PLC boolean read Tags"."AT in sunshad wand lower pos"."DataSocket Reference"."OnDataUpdated" format="%.0x"; "PLC Comms"."PLC boolean read Tags"."AT in glass wand lower pos"."DataSocket Reference"."OnStatusUpdated" format="%.0x"; "PLC Comms"."PLC boolean read Tags"."AT in glass wand lower pos"."DataSocket Reference"."OnDataUpdated" format="%.0x"; "PLC Comms"."PLC boolean read Tags"."AT shade position"."DataSocket Reference"."OnStatusUpdated" format="%.0x"; "PLC Comms"."PLC boolean read Tags"."AT shade position"."DataSocket Reference"."OnDataUpdated" format="%.0x"; "PLC Comms"."PLC boolean read Tags"."AT glass position"."DataSocket Reference"."OnStatusUpdated" format="%.0x"; "PLC Comms"."PLC boolean read Tags"."AT glass position"."DataSocket Reference"."OnDataUpdated" format="%.0x"; "Store Data"."Sun Shade Open Force Limits"."Variance" format="%.2g"; "Store Data"."Sun Shade Open Force Limits"."Truncation End" format="%.2g"; "Store Data"."Sun Shade Open Force Limits"."Truncation Start" format="%.2g"; "Store Data"."Sun Shade Open Force Limits"."Avg Max" format="%.2g"; "Store Data"."Sun Shade Open Force Limits"."Avg Min" format="%.2g"; "Store Data"."Sun Shade Open Force Limits"."Overall Max" format="%.2g"; "Store Data"."Sun Shade Open Force Limits"."Overall Min" format="%.2g"; "Store Data"."Sun Shade Close Force Limits"."Variance" format="%.2g"; "Store Data"."Sun Shade Close Force Limits"."Truncation End" format="%.2g"; "Store Data"."Sun Shade Close Force Limits"."Truncation Start" format="%.2g"; "Store Data"."Sun Shade Close Force Limits"."Avg Max" format="%.2g"; "Store Data"."Sun Shade Close Force Limits"."Avg Min" format="%.2g"; "Store Data"."Sun Shade Close Force Limits"."Overall Max" format="%.2g"; "Store Data"."Sun Shade Close Force Limits"."Overall Min" format="%.2g"}, 11 "hmi status indicator ref":refnum<vi>) -> (0 "error out":errorcluster)   [LabVIEW 2018]
uses:
  <vilib>/Instr/_visa.llb/VISA Configure Serial Port (Instr).vi
  05.UserVI's/BarCode/typedefs/barcode printer types.ctl
  05.UserVI's/BarCode/typedefs/barcode format params.ctl
  05.UserVI's/type defs/EOL Motor Type.ctl
  05.UserVI's/type defs/RAP Signal Control.ctl
  05.UserVI's/type defs/Communication with Motors.ctl
  02.Type Def's/All Communication Types.ctl
  05.UserVI's/type defs/EOL Part Setup.ctl
  02.Type Def's/All Motions.ctl
  02.Type Def's/EOL Switch Max Min Check Cluster.ctl
  02.Type Def's/EOL Switch Value Configuration Cluster.ctl
  02.Type Def's/All Switch Configuration Cluster.ctl
  05.UserVI's/type defs/17x Sunshade Limts Seq.ctl
  02.Type Def's/Pass Fail Control.ctl
  02.Type Def's/EOL Module Info Control.ctl
  05.UserVI's/type defs/17x AP Data Type.ctl
  05.UserVI's/type defs/17x Audit Motion Data Seq Control.ctl
  02.Type Def's/EOL Motion Database Table.ctl
  05.UserVI's/sequence/type defs/Sequence Info.ctl
  02.Type Def's/station nvh config.ctl
  05.UserVI's/type defs/EOL Global Digital Output Control.ctl
  02.Type Def's/station DO map.ctl
  02.Type Def's/station rs232 port map.ctl
  02.Type Def's/station ethernet address map.ctl
  02.Type Def's/station paths.ctl
  <vilib>/Platform/dataskt.llb/DataSocket Reference Type.ctl
  05.UserVI's/type defs/plc path and tag.ctl
  02.Type Def's/station plc read boolean tags.ctl
  02.Type Def's/EOL Save Module Test Data Control.ctl
  05.UserVI's/type defs/EOL Global Digital Input Control.ctl
  02.Type Def's/station DI map.ctl
  02.Type Def's/station plc read string tags.ctl
  02.Type Def's/station plc write boolean tags.ctl
  02.Type Def's/station plc write string tags.ctl
  02.Type Def's/Screen Motion Data.ctl
  02.Type Def's/station motion data indicator.ctl
  02.Type Def's/lvdt name val pair.ctl
  02.Type Def's/station hmi.ctl
  02.Type Def's/individual station status.ctl
  02.Type Def's/control refs.ctl
  05.UserVI's/type defs/EOL LVDT's Check Controller.ctl
  05.UserVI's/Lambda Power/power supply types.ctl
  05.UserVI's/LVDT's/lvdt precision.ctl
  02.Type Def's/main state cluster.ctl
  02.Type Def's/station plc read float tags.ctl
  02.Type Def's/plc comms params.ctl
  02.Type Def's/iGPS float tags.ctl
  02.Type Def's/sequence state.ctl
  03.Inalfa LIN/LIN Device.ctl
  <vilib>/CMC.AME/Inalfa ADCS/Ctl'Def/ADCS_LIN info.ctl
  C:/Program Files (x86)/National Instruments/LabVIEW 2018/vi.lib/CMC.AME/_Inalfa TS LIN_internal_deps/Interop.TSMasterAPI.dll
  Program Files (x86)/National Instruments/LabVIEW 2018/vi.lib/CMC.AME/_Inalfa TS LIN_internal_deps/Interop.TSMasterAPI.dll
  02.Type Def's/station LIN config.ctl
  02.Type Def's/misc station config.ctl
panel:
  # "start/abort only used by barcode instance, since there are discrete signals for this in the other stations."
  # "Sunroof Barcode"
  # "Pallet Number"
  # "Part Type"
  # "Application Status"
  # "Current Step"
  # "Cycle Time"
  # "Pass / Fail"
  # "Shade Close"
  # "Actual Data"
  # "Limits"
  # "Avg Current"
  # "Run Time"
  # "Speed"
  # "Noise Test"
  # "Position"
  # "Shade Open"
  # "Actual Data"
  # "Limits"
  # "Avg Current"
  # "Run Time"
  # "Speed"
  # "Noise Test"
  # "Position"
  # "Vent Close"
  # "Actual Data"
  # "Limits"
  # "Avg Current"
  # "Run Time"
  # "Speed"
  # "Noise Test"
  # "Position"
  # "Vent Open"
  # "Actual Data"
  # "Limits"
  # "Avg Current"
  # "Run Time"
  # "Speed"
  # "Noise Test"
  # "Position"
  # "Slide Close"
  # "Actual Data"
  # "Limits"
  # "Avg Current"
  # "Run Time"
  # "Speed"
  # "Noise Test"
  # "Position"
  # "Slide Open"
  # "Actual Data"
  # "Limits"
  # "Avg Current"
  # "Run Time"
  # "Speed"
  # "Noise Test"
  # "Position"
  # "Min"
  # "N"
  # "Min"
  # "Start"
  # "N"
  # "Max"
  # "N"
  # "Max"
  # "N"
  # "End"
  # "Min"
  # "N"
  # "Min"
  # "Start"
  # "N"
  # "Max"
  # "N"
  # "Max"
  # "N"
  # "End"
  # "Min"
  # "Max"
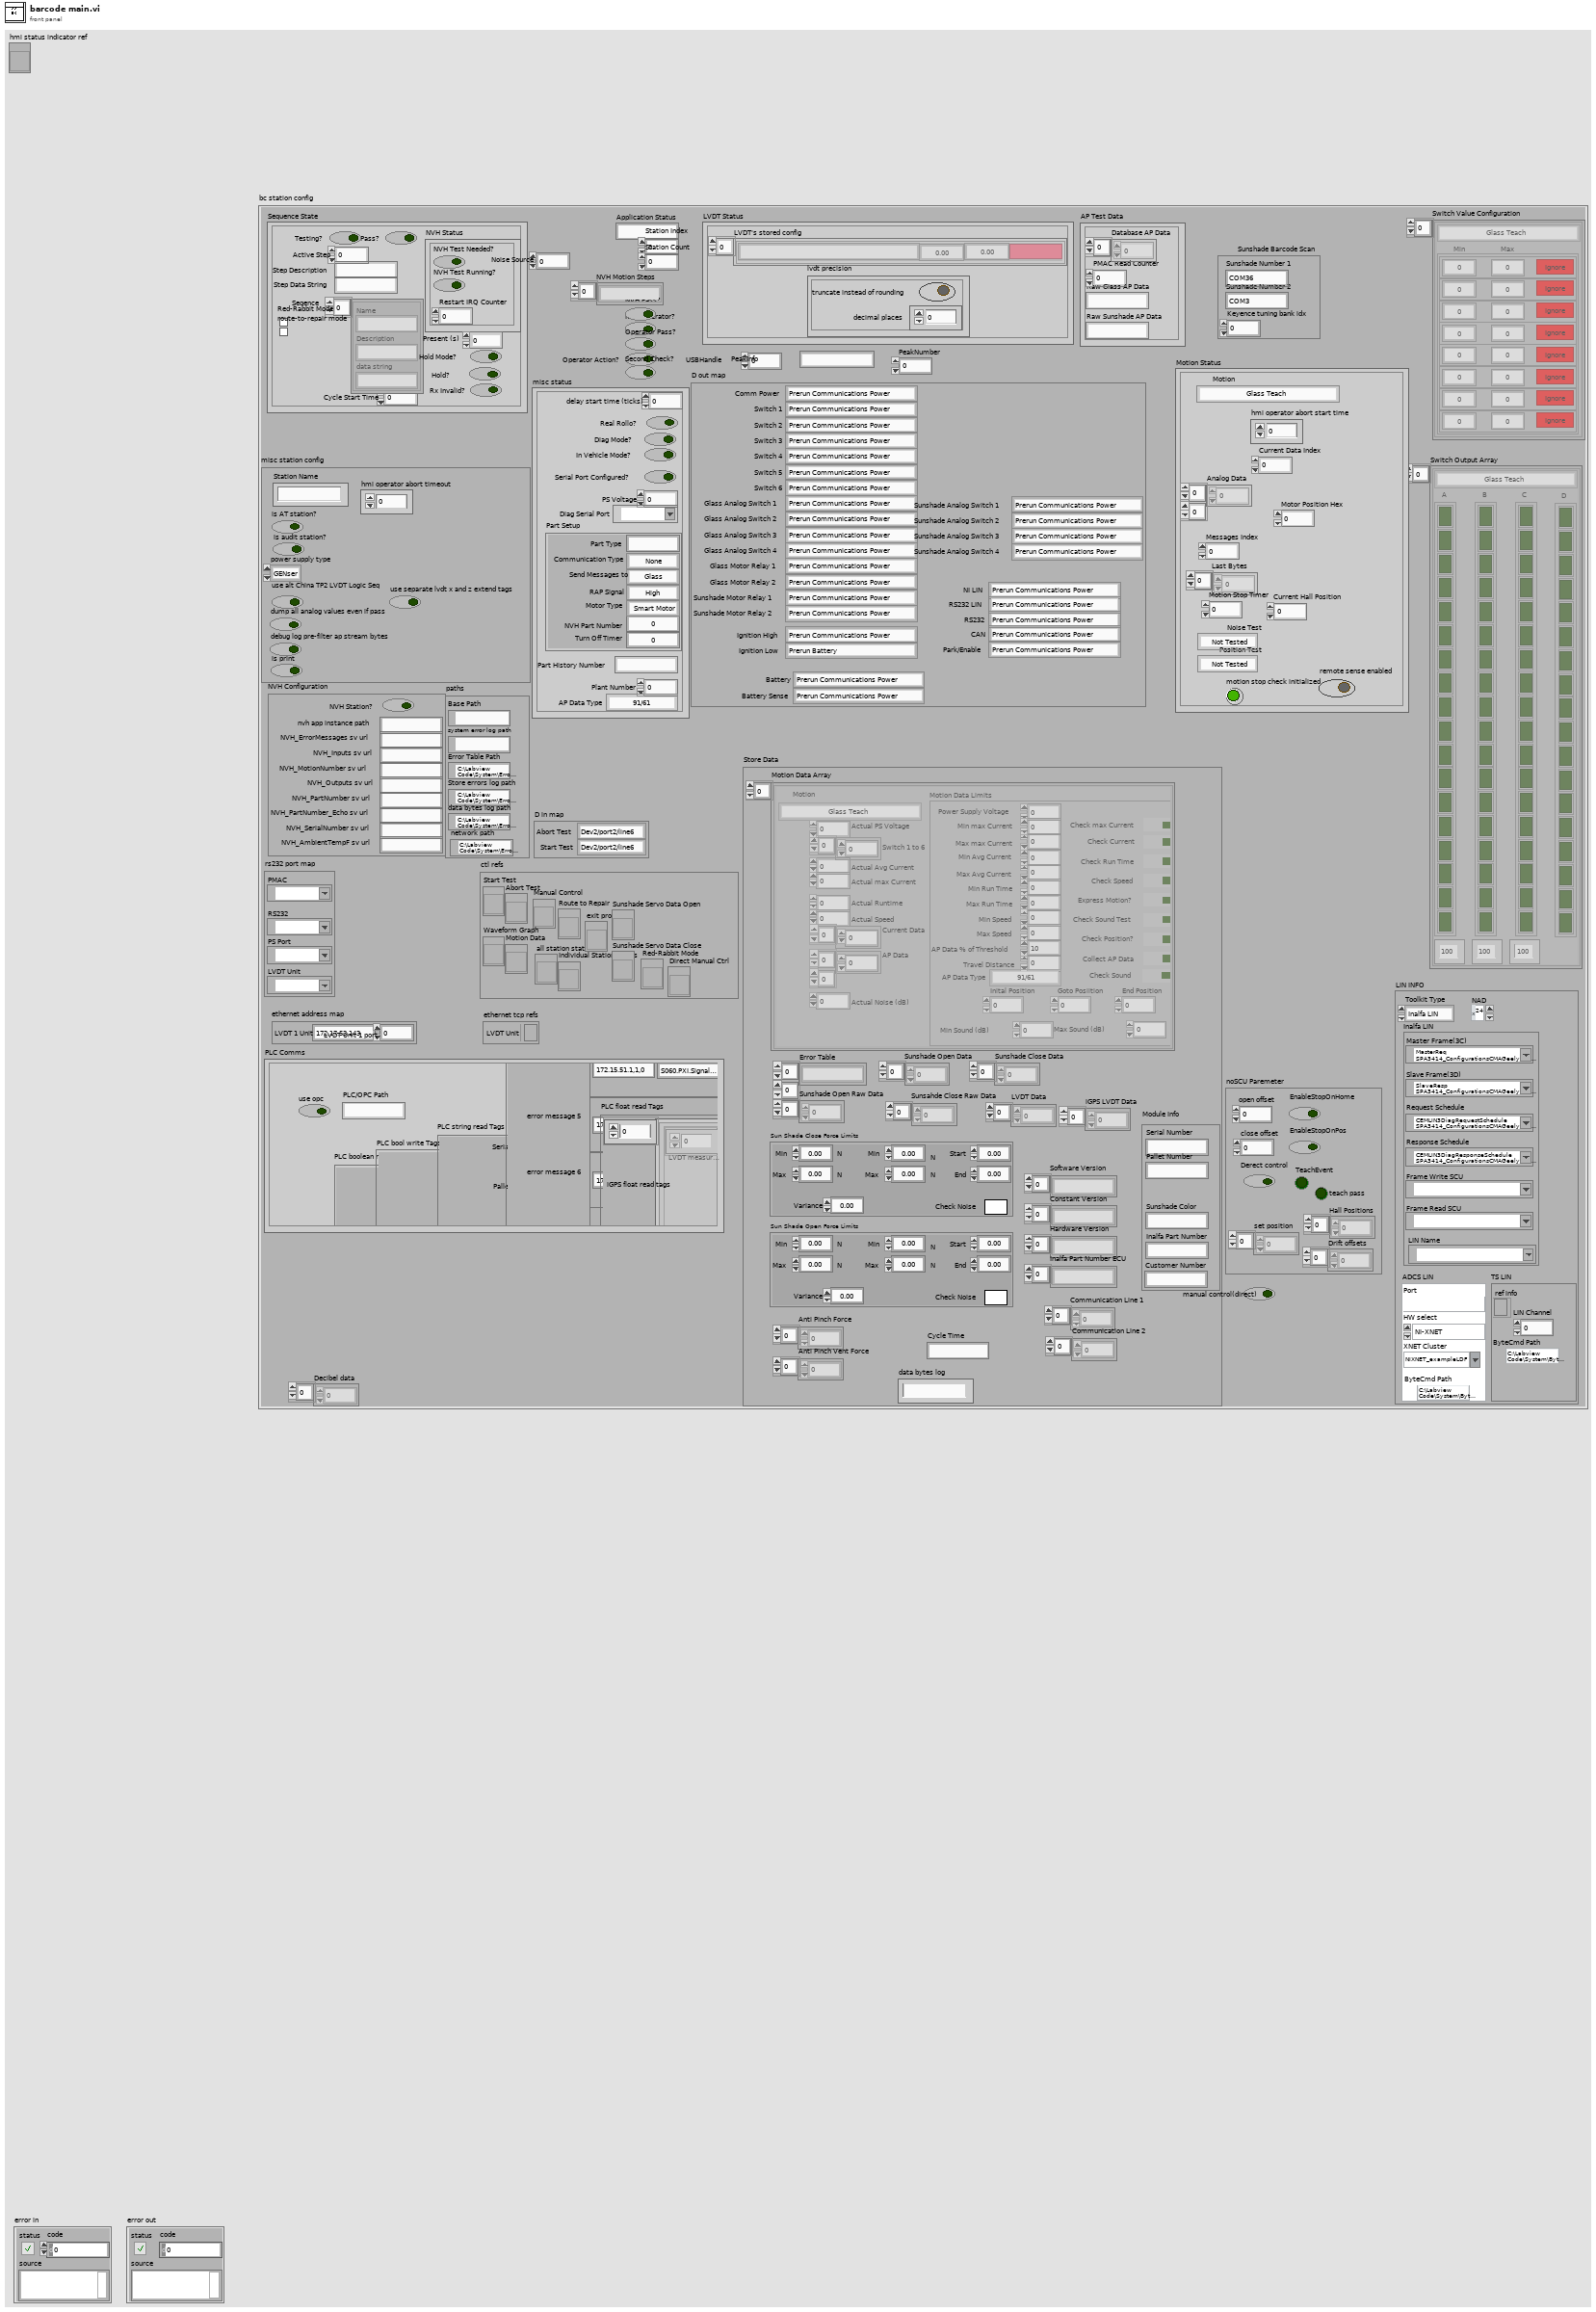
[diagram p1: front panel]
types:
  T1 = typedef "main state cluster.ctl" = cluster{"Application Status":string, "Switch Output Array":T2[], "Switch Value Configuration":T4[], "NVH Configuration":T6, "D out map":T7, "rs232 port map":T9, "ethernet address map":T10, "paths":T11, "Station Index":i32, "Station Count":i32, "Store Data":T12, "D in map":T18, "ctl refs":T20, "misc station config":T21, "ethernet tcp refs":cluster{"LVDT Unit":refnum<k5>}, "PLC Comms":T23, "Sunshade Barcode Scan":cluster{"Sunshade Number 2":string, "Sunshade Number 1":string, "Keyence tuning bank idx":i32}, "AP Test Data":cluster{"Raw Sunshade AP Data":string, "Raw Glass AP Data":string, "PMAC Read Counter":dbl, "Database AP Data":dbl[]}, "Motion Status":cluster{"hmi operator abort start time":u32, "Current Data Index":i32, "Analog Data":sgl[][], "Motor Position Hex":u16, "Messages Index":u16, "Last Bytes":u8[], "Current Hall Position":i16, "Motion Stop Timer":u32, "Position Test":T32, "Noise Test":T32, "motion stop check initialized":bool, "remote sense enabled":bool, "Motion":T3}, "LVDT Status":cluster{"LVDT's stored config":T33[], "lvdt precision":T34}, "Sequence State":T35, "misc status":cluster{"delay start time (ticks)":u32, "In Vehicle Mode?":bool, "Diag Mode?":bool, "Serial Port Configured?":bool, "PS Voltage":dbl, "Diag Serial Port":refnum<visa-resource-name>, "Part Setup":T37, "Part History Number":string, "Plant Number":u8, "AP Data Type":T15, "Real Rollo?":bool}, "NVH Operator?":bool, "NVH Pass?":bool, "Operator Pass?":bool, "Operator Action?":bool, "Noise Source":u32, "USBHandle":i32, "PeakInfo":string, "PeakNumber":i32, "NVH Motion Steps":string[], "Second Check?":bool, "Decibel data":dbl[], "noSCU Paremeter":cluster{"EnableStopOnHome":bool, "EnableStopOnPos":bool, "TeachEvent":bool, "open offset":i32, "close offset":i32, "Derect control":bool, "set position":i32[], "teach pass ":bool, "Drift offsets":i32[], "Hall Positions":i32[]}, "manual control(direct)":bool, "LIN INFO":T42}
  T2 = typedef "All Switch Configuration Cluster.ctl" = cluster{"All Motions":T3, "A":bool[], "B":bool[], "C":bool[], "D":bool[], "A activation time (ms)":u32, "B activation time (ms)":u32, "C activation time (ms)":u32}
  T3 = typedef "All Motions.ctl" = enum16{"Glass Teach", "Glass Slide Open", "Glass Slide Close", "Glass Vent Open", "Glass Vent Close", "Sunshade Teach", "Sunshade Open", "Sunshade Close", "Idle", "Sunshade Open 2", "Sunshade Close 2", "Glass Slide Open Sunshade Open", "Glass Slide Open Sunshade Close", "Glass Slide Close Sunshade Open", "Glass Slide Close Sunshade Close", "Glass Vent Open Sunshade Open", "Glass Vent Open Sunshade Close", "Glass Vent Close Sunshade Open", "Glass Vent Close Sunshade Close", "Express Glass Slide Open", "Express Glass Slide Close", "Express Glass Vent Open", "Express Glass Vent Close", "Express Sunshade Open", "Express Sunshade Close", "Express Sunshade Open 2", "Express Sunshade Close 2", "Express Glass Slide Open Sunshade Open", "Express Glass Slide Open Sunshade Close", "Express Glass Slide Close Sunshade Open", "Express Glass Slide Close Sunshade Close", "Express Glass Vent Open Sunshade Open", "Express Glass Vent Open Sunshade Close", "Express Glass Vent Close Sunshade Open", "Express Glass Vent Close Sunshade Close", "Goto Position Glass", "Goto Position Sunshade", "Sunshade Teach 2"}
  T4 = typedef "EOL Switch Value Configuration Cluster.ctl" = cluster{"All Motions":T3, "Array":T5[]}
  T5 = typedef "EOL Switch Max Min Check Cluster.ctl" = cluster{"Min":dbl, "Max":dbl, "Check?":bool}
  T6 = typedef "station nvh config.ctl" = cluster{"NVH Station?":bool, "nvh app instance path":string, "NVH_ErrorMessages sv url":string, "NVH_Inputs sv url":string, "NVH_MotionNumber sv url":string, "NVH_Outputs sv url":string, "NVH_PartNumber sv url":string, "NVH_PartNumber_Echo sv url":string, "NVH_SerialNumber sv url":string, "NVH_AmbientTempF sv url":string}
  T7 = typedef "station DO map.ctl" = cluster{"Comm Power":T8, "Switch 1":T8, "Switch 2":T8, "Switch 3":T8, "Switch 4":T8, "Switch 5":T8, "Switch 6":T8, "Glass Analog Switch 1":T8, "Glass Analog Switch 2":T8, "Glass Analog Switch 3":T8, "Glass Analog Switch 4":T8, "Glass Motor Relay 1":T8, "Glass Motor Relay 2":T8, "Sunshade Motor Relay 1":T8, "Sunshade Motor Relay 2":T8, "Ignition High":T8, "Ignition Low":T8, "Battery":T8, "Sunshade Analog Switch 1":T8, "Sunshade Analog Switch 2":T8, "Sunshade Analog Switch 3":T8, "Sunshade Analog Switch 4":T8, "NI LIN":T8, "RS232 LIN":T8, "RS232":T8, "CAN":T8, "Park/Enable":T8, "Battery Sense":T8}
  T8 = typedef "EOL Global Digital Output Control.ctl" = enum16{"Prerun Battery", "Prerun Ignition High", "Prerun Switch 1", "Prerun Switch 2", "Prerun Switch 3", "Prerun Select NI LIN", "Prerun Switch 4", "Prerun Switch 5", "Prerun Switch 6", "Prerun Ignition Low", "Prerun Glass Analog Switch 1", "Prerun Glass Analog Switch 2", "Prerun Glass Analog Switch 3", "Prerun Glass Analog Switch 4", "Prerun Sunshade Analog Switch 1", "Prerun Sunshade Analog Switch 2", "Prerun Sunshade Analog Switch 3", "Prerun Sunshade Analog Switch 4", "Prerun Select RS232 LIN", "Prerun Select RS232", "Prerun Select CAN", "Prerun Park/Enable", "Prerun Communications Power", "Prerun BMW Glass Motor Relay 1", "Prerun BMW Glass Motor Relay 2", "Prerun BMW Sunshade Motor Relay 1", "Prerun BMW Sunshade Motor Relay 2", "Prerun Spare 1", "Prerun Spare 2", "Prerun Spare 3", "Prerun Spare 4", "Prerun Spare 5", "Audit Battery", "Audit Ignition High", "Audit Ignition Low", "Audit Switch 1", "Audit Switch 2", "Audit Switch 3", "Audit Switch 4", "Audit Switch 5", "Audit Switch 6", "Audit Glass Analog Switch 1", "Audit Glass Analog Switch 2", "Audit Glass Analog Switch 3", "Audit Glass Analog Switch 4", "Audit Sunshade Analog Switch 1", "Audit Sunshade Analog Switch 2", "Audit Sunshade Analog Switch 3", "Audit Sunshade Analog Switch 4", "Audit Select NI LIN", "Audit Select RS232 LIN", "Audit Select RS232", "Audit Select CAN", "Audit Park/Enable", "Audit Communications Power", "Audit BMW Glass Motor Relay 1", "Audit BMW Glass Motor Relay 2", "Audit BMW Sunshade Motor Relay 1", "Audit BMW Sunshade Motor Relay 2", "Audit Spare 1", "Audit Spare 2", "Audit Spare 3", "Audit Spare 4", "Audit Spare 5", "Repair Battery", "Repair Ignition High", "Repair Switch 1", "Repair Switch 2", "Repair Select NI LIN", "Repair Ignition Low", "Repair Switch 3", "Repair Switch 4", "Repair Switch 5", "Repair Switch 6", "Repair Glass Analog Switch 1", "Repair Glass Analog Switch 2", "Repair Glass Analog Switch 3", "Repair Glass Analog Switch 4", "Repair Sunshade Analog Switch 1", "Repair Sunshade Analog Switch 2", "Repair Sunshade Analog Switch 3", "Repair Sunshade Analog Switch 4", "Repair Select RS232 LIN", "Repair Select RS232", "Repair Select CAN", "Repair Select Park/Enable", "Repair Communications Power", "Repair BMW Glass Motor Relay 1", "Repair BMW Glass Motor Relay 2", "Repair BMW Sunshade Motor Relay 1", "Repair BMW Sunshade Motor Relay 2", "Repair Spare 1", "Repair Spare 2", "Repair Spare 3", "Repair Spare 4", "Repair Spare 5", "Breakin Battery", "Breakin Igntiion High", "Breakin Ignition Low", "Breakin Switch 1", "Breakin Switch 2", "Breakin Switch 3", "Breakin Switch 4", "Breakin Switch 5", "Breakin Switch 6", "Breakin Glass Analog Switch 1", "Breakin Glass Analog Switch 2", "Breakin Glass Analog Switch 3", "Breakin Glass Analog Switch 4", "Breakin Sunshade Analog Switch 1", "Breakin Sunshade Analog Switch 2", "Breakin Sunshade Analog Switch 3", "Breakin Sunshade Analog Switch 4", "Breakin Select NI LIN", "Breakin Select RS232 LIN", "Breakin Select RS232", "Breakin Select CAN", "Breakin Park/Enable", "Breakin Communications Power", "Breakin BMW Glass Motor Relay 1", "Breakin BMW Glass Motor Relay 2", "Breakin BMW Sunshade Motor Relay 1", "Breakin BMW Sunshade Motor Relay 2", "Breakin Spare 1", "Breakin Spare 2", "Breakin Spare 3", "Breakin Spare 4", "Breakin Spare 5", "Not Implemented"}
  T9 = typedef "station rs232 port map.ctl" = cluster{"PMAC":refnum<visa-resource-name>, "PS Port":refnum<visa-resource-name>, "LVDT Unit":refnum<visa-resource-name>, "RS232":refnum<visa-resource-name>}
  T10 = typedef "station ethernet address map.ctl" = cluster{"LVDT 1 Unit":string, "LVDT Unit 1 port":u16}
  T11 = typedef "station paths.ctl" = cluster{"Base Path":path, "system error log path":path, "Error Table Path":path, "Store errors log path":path, "data bytes log path":path, "network path":path}
  T12 = typedef "EOL Save Module Test Data Control.ctl" = cluster{"Motion Data Array":T13[], "Error Table":string[][], "Sun Shade Close Force Limits":T16, "Sun Shade Open Force Limits":T16, "Sunshade Open Data":sgl[], "Sunshade Close Data":sgl[], "Module Info":T17, "Sunsahde Close Raw Data":sgl[], "Sunshade Open Raw Data":sgl[], "Software Version":string[], "Constant Version":string[], "Hardware Version":string[], "Inalfa Part Number ECU":string[], "LVDT Data":sgl[], "Communication Line 1":sgl[], "Communication Line 2":sgl[], "Anti Pinch Force":sgl[], "Cycle Time":string, "Anti Pinch Vent Force":sgl[], "iGPS LVDT Data":sgl[], "data bytes log":string}
  T13 = typedef "EOL Motion Database Table.ctl" = cluster{"Motion":T3, "Actual Avg Current":dbl, "Actual Runtime":dbl, "Actual Speed":dbl, "Current Data":sgl[], "Motion Data Limits":T14, "Switch 1 to 6":dbl[], "Actual PS Voltage":dbl, "AP Data":i16[][], "Actual max Current":dbl, "Actual Noise (dB)":dbl}
  T14 = typedef "17x Audit Motion Data Seq Control.ctl" = cluster{"Power Supply Voltage":dbl, "Min Avg Current":dbl, "Max Avg Current":dbl, "Min Run Time":dbl, "Max Run Time":dbl, "Min Speed":dbl, "Max Speed":dbl, "AP Data % of Threshold":dbl, "Travel Distance":dbl, "AP Data Type":T15, "Check Current":bool, "Check Run Time":bool, "Check Speed":bool, "Express Motion?":bool, "Check Sound Test":bool, "Check Position?":bool, "Collect AP Data":bool, "Inital Position":u16, "End Position":u16, "Goto Posiition":u16, "Max max Current":dbl, "Min max Current":dbl, "Check max Current":bool, "Check Sound":bool, "Min Sound (dB)":dbl, "Max Sound (dB)":dbl}
  T15 = typedef "17x AP Data Type.ctl" = enum16{"91/61", "92/62", "93/63", "67", "68", "6F", "71", "91 Msg", "92 Msg", "93 Msg", "94 Msg", "HiRain 91", "HiRain 92 Speed", "HiRain 92 HS", "HiRain 92", "HiRain 93", "SnT"}
  T16 = typedef "17x Sunshade Limts Seq.ctl" = cluster{"Overall Min":dbl, "Overall Max":dbl, "Avg Min":dbl, "Avg Max":dbl, "Truncation Start":dbl, "Truncation End":dbl, "Variance":dbl, "Check Noise":bool}
  T17 = typedef "EOL Module Info Control.ctl" = cluster{"Serial Number":string, "Pallet Number":string, "Sunshade Color":string, "Inalfa Part Number":string, "Customer Number":string}
  T18 = typedef "station DI map.ctl" = cluster{"Abort Test":T19, "Start Test":T19}
  T19 = typedef "EOL Global Digital Input Control.ctl" = enum16{"Dev2/port0/line0", "Dev2/port0/line1", "Dev2/port0/line2", "Dev2/port0/line3", "Dev2/port0/line4", "Dev2/port0/line5", "Dev2/port0/line6", "Dev2/port0/line7", "Dev2/port1/line0", "Dev2/port1/line1", "Dev2/port1/line2", "Dev2/port1/line3", "Dev2/port1/line4", "Dev2/port1/line5", "Dev2/port1/line6", "Dev2/port1/line7", "Dev2/port2/line0", "Dev2/port2/line1", "Dev2/port2/line2", "Dev2/port2/line3", "Dev2/port2/line4", "Dev2/port2/line5", "Dev2/port2/line6", "Dev2/port2/line7", "Prerun Start Test", "Prerun Abort Test", "Audit Start Test", "Audit Abort Test", "Dev2/port3/line4", "Dev2/port3/line5", "Breakin Start Test", "Breakin Abort Test", "Not Implemented"}
  T20 = typedef "control refs.ctl" = cluster{"Start Test":refnum<vi>, "Abort Test":refnum<vi>, "Manual Control":refnum<vi>, "Route to Repair":refnum<vi>, "Waveform Graph":refnum<vi>, "Motion Data":refnum<vi>, "all station status":refnum<vi>, "Individual Station Status":refnum<vi>, "exit program":refnum<vi>, "Sunshade Servo Data Open":refnum<vi>, "Sunshade Servo Data Close":refnum<vi>, "Red-Rabbit Mode":refnum<vi>, "Direct Manual Ctrl":refnum<vi>}
  T21 = typedef "misc station config.ctl" = cluster{"Station Name":string, "is AT station?":bool, "is audit station?":bool, "power supply type":T22, "use alt China TP2 LVDT Logic Seq":bool, "hmi operator abort timeout":u32, "dump all analog values even if pass":bool, "debug log pre-filter ap stream bytes":bool, "use separate lvdt x and z extend tags":bool, "is print":bool}
  T22 = typedef "power supply types.ctl" = enum16{"GENser", "ZUPser", "GENeth", "Manual", "ITECH"}
  T23 = typedef "plc comms params.ctl" = cluster{"PLC boolean read Tags":T24, "PLC bool write Tags":T27, "PLC string read Tags":T28, "PLC string write Tags":T29, "use opc":bool, "PLC/OPC Path":string, "PLC float read Tags":T30}
  T24 = typedef "station plc read boolean tags.ctl" = cluster{"AT glass position":T25, "AT shade position":T25, "AT in glass wand lower pos":T25, "AT in sunshad wand lower pos":T25, "AT in wand home pos":T25, "LVDT's Extended":T25, "motor foam present LH":T25, "motor foam present RH":T25, "audit gap hider present LH":T25, "audit gap hider present RH":T25, "FB light block present":T25, "bolt check 1":T25, "bolt check 2":T25, "bolt check 3":T25, "bolt check 4":T25, "bolt check 5":T25, "bolt check 6":T25, "bolt check 7":T25, "bolt check 8":T25, "bolt check 9":T25, "bolt check 10":T25, "bolt check 11":T25, "bolt check 12":T25, "bolt check 13":T25, "bolt check 14":T25, "bolt check 15":T25, "bolt check 16":T25, "bolt check 17":T25, "bolt check 18":T25, "bolt check 19":T25, "bolt check 20":T25, "bolt check 21":T25, "start":T25, "abort":T25, "LVDT's Retracted":T25, "manual barcode print":T25, "ss servo at open":T25, "ss servo at close":T25, "ss servo opening":T25, "ss servo closing":T25, "control slide at home":T25, "control slide left good":T25, "control slide left over stroke":T25, "control slide right good":T25, "control slide right over stroke":T25, "wind deflector high speed pos":T25, "wind deflector low speed pos":T25, "AT VentPMACatHome":T25, "AT VentPMACisExtend":T25, "SS Barcode Scanner Bypassed":T25, "Check Frame Barcode":T25, "iGPS Pass 0":T25, "iGPS Pass 1":T25, "iGPS Pass 2":T25, "iGPS Pass 3":T25, "iGPS Pass 4":T25, "iGPS Pass 5":T25, "iGPS Pass 6":T25, "iGPS Pass 7":T25, "iGPS Pass 8":T25, "iGPS Pass 9":T25, "Z LVDTs Extended":T25, "NVH Operator Pass":T25, "NVH Operator Fail":T25, "NVH Operator Express Glass Open":T25, "NVH Operator Express Glass Close":T25, "NVH Operator Express Rollo Open01":T25, "NVH Operator Express Rollo Close01":T25, "NVH Operator Express Rollo Open02":T25, "NVH Operator Express Rollo Close02":T25, "NVH Operator Vent Open Noise":T25, "NVH Operator Vent Close Noise":T25, "NVH Operator Sunshade Open Noise":T25, "NVH Operator Sunshade Close Noise":T25, "NVH Operator Glass Open Noise":T25, "NVH Operator Glass Close Noise":T25, "NVH Operator Finish":T25, "NVH Operator Check":T25, "AT shade 02 position":T25, "AT in sunshad 02 wand up pos":T25, "AT in wand 02 home pos":T25, "windproof position":T25, "NVH Operator Express Glass vent Open":T25, "NVH Operator Express Glass Vent Close":T25, "NVH Operator Re-do":T25, "AT at vent ATS test pos":T25, "AT at vent ATS Home pos":T25, "Start Adjust LVDT":T25, "Finish Adjust LVDT":T25}
  T25 = typedef "plc path and tag.ctl" = cluster{"Tag Name":string, "Network Path":string, "use opc":bool, "DataSocket Reference":T26}
  T26 = typedef "DataSocket Reference Type.ctl" = cluster{"CWDSLib._DCWDataSocket":refnum<k7>, "CWDSLib._DCWData":refnum<k7>, "OnDataUpdated":u32, "OnStatusUpdated":u32}
  T27 = typedef "station plc write boolean tags.ctl" = cluster{"AT set glass wand lower":T25, "AT set sunshade wand lower":T25, "AT set wand home pos":T25, "Test Complete Pass":T25, "Test Complete Fail":T25, "Test Started":T25, "Retract LVDT's":T25, "Extend LVDT's":T25, "ss servo open":T25, "ss servo close":T25, "control slide start":T25, "control slide stop":T25, "AT VentPMACHome":T25, "AT VentPMACExtended":T25, "Good Frame Barcode":T25, "Bad Frame Barcode":T25, "Extend Z LVDTS":T25, "NVH SunRoof Moving":T25, "NVH SunRoof Stop":T25, "NVH Pass":T25, "NVH Fail":T25, "NVH Operator Express Glass Opened":T25, "NVH Operator Express Glass Closed":T25, "NVH Operator Express Rollo Opened01":T25, "NVH Operator Express Rollo Closed01":T25, "NVH Operator Express Rollo Opened02":T25, "NVH Operator Pass":T25, "NVH Operator Fail":T25, "NVH Operator Check":T25, "NVH Operator Vent Open Noise":T25, "NVH Operator Vent Close Noise":T25, "NVH Operator Sunshade Open Noise":T25, "NVH Operator Sunshade Close Noise":T25, "NVH Operator Glass Open Noise":T25, "NVH Operator Glass Close Noise":T25, "NVH Operator Finish":T25, "AT set sunshade 02 wand up":T25, "AT set wand 02 home pos":T25, "Barcode01 OK":T25, "Barcode02 OK":T25, "AT set to Vent ATS Test Pos":T25, "AT set to Vent ATS Home Pos":T25, "Move LVDT Adjust Station":T25}
  T28 = typedef "station plc read string tags.ctl" = cluster{"Serial Number":T25, "Pallet Number":T25, "Inalfa Part Number":T25, "Shade Color":T25, "Model Type":T25, "Customer Number":T25, "Part History Number":T25, "Shade 1 Barcode":T25, "Shade 2 Barcode":T25, "Manual Serial Number":T25, "Manual Inalfa Part Number":T25, "Manual Shade Color":T25, "Manual Model Type":T25, "Manual Customer Number":T25, "Manual Part History Number":T25, "iGPS SN 0":T25, "iGPS SN 1":T25, "iGPS SN 2":T25, "iGPS SN 3":T25, "iGPS SN 4":T25, "iGPS SN 5":T25, "iGPS SN 6":T25, "iGPS SN 7":T25, "iGPS SN 8":T25, "iGPS SN 9":T25}
  T29 = typedef "station plc write string tags.ctl" = cluster{"barcode station error":T25, "error message 0":T25, "error message 1":T25, "error message 2":T25, "error message 3":T25, "error message 4":T25, "error message 5":T25, "error message 6":T25, "error message 7":T25, "error message 8":T25, "error message 9":T25}
  T30 = typedef "station plc read float tags.ctl" = cluster{"iGPS float read tags":T31[]}
  T31 = typedef "iGPS float tags.ctl" = cluster{"LVDT measurements":cluster{"value":T25, "UCL":T25, "LCL":T25, "LVDT Name":string}[]}
  T32 = typedef "Pass Fail Control.ctl" = enum16{"Not Tested", "Pass", "Fail"}
  T33 = typedef "EOL LVDT's Check Controller.ctl" = cluster{"Upper Limit":dbl, "Lower Limit":dbl, "LVDT Name":string, "Check":bool}
  T34 = typedef "lvdt precision.ctl" = cluster{"truncate instead of rounding":bool, "decimal places":u8}
  T35 = typedef "sequence state.ctl" = cluster{"Step Description":string, "Cycle Start Time":u32, "Step Data String":string, "Pass?":bool, "Seqence":T36[], "Active Step":u8, "Testing?":bool, "Red-Rabbit Mode":bool, "route-to-repair mode":bool, "NVH Status":cluster{"Restart IRQ Counter":u8, "NVH Test Needed?":bool, "NVH Test Running?":bool}, "Present (s)":dbl, "Hold Mode?":bool, "Hold?":bool, "Rx Invalid?":bool}
  T36 = typedef "Sequence Info.ctl" = cluster{"Name":string, "Description":string, "data string":string}
  T37 = typedef "EOL Part Setup.ctl" = cluster{"Communication Type":T38, "Send Messages to":T39, "RAP Signal":T40, "Motor Type":T41, "NVH Part Number":u16, "Turn Off Timer":u16, "Part Type":string}
  T38 = typedef "All Communication Types.ctl" = enum16{"None", "CAN", "RS 232", "RS 232 LIN", "GM LIN", "SnT LIN", "K Line", "Robel CAN", "P42M-Continental", "Inalfa SCU LIN", "Spare 3"}
  T39 = typedef "Communication with Motors.ctl" = enum16{"Glass", "Rollo", "Both"}
  T40 = typedef "RAP Signal Control.ctl" = enum16{"High", "Low", "None"}
  T41 = typedef "EOL Motor Type.ctl" = enum16{"Smart Motor", "Sensor Motor"}
  T42 = typedef "station LIN config.ctl" = cluster{"Toolkit Type":enum16{"Inalfa LIN", "ADCS LIN", "TS LIN"}, "NAD":u8, "Inalfa LIN":T43, "ADCS LIN":T44, "TS LIN":cluster{"ref info":refnum<k24>, "LIN Channel":i32, "ByteCmd Path":path}}
  T43 = typedef "LIN Device.ctl" = cluster{"Master Frame(3C)":refnum<k21>, "Slave Frame(3D)":refnum<k21>, "Request Schedule":refnum<k21>, "Response Schedule":refnum<k21>, "Frame Write SCU":refnum<k21>, "Frame Read SCU":refnum<k21>, "LIN Name":refnum<k21>}
  T44 = typedef "ADCS_LIN info.ctl" = cluster{"Port":string, "HW select":u16, "XNET Cluster":string, "ByteCmd Path":path}
  T45 = typedef "barcode format params.ctl" = cluster{"Format String":string, "Print String":string, "Quantity":u8, "printer type":T46, "RS232 Port":string, "IP Address":string, "Ethernet Port":u32}
  T46 = typedef "barcode printer types.ctl" = enum16{"Intermec RS232", "Intermec Ethernet"}
  T47 = cluster{"Frame Barcode Formats":T45[], "SS Barcode Reader":refnum<visa-resource-name>, "Serial Number":string, "Barcode Data 1":string, "Inalfa Part Number":string, "Error Message":string, "Color":string, "PLC Barcode Data 1":string, "Start Test":bool, "Model Type":string, "Barcode Data 2":string, "Start Timer":dbl, "PHN":string, "PLC Barcode Data 2":string, "Customer Number":string, "SS barcode scanner ip":string, "PLC boolean read Tags":T24, "PLC string read Tags":T28, "PLC bool write Tags":T27, "PLC string write Tags":T29, "Base Path":path, "hmi status indicator ref":refnum<vi>, "Manual Control":refnum<vi>, "exit program":refnum<vi>}
  T48 = typedef "barcode station status.ctl" = cluster{"Customer Number":string, "PHN":string, "PLC Barcode Data 2":string, "Test Running":bool, "Station Application Status":string, "Scanner Data 1":string, "PLC Barcode Data 1":string, "PLC Info":string, "Model Type":string, "Color":string, "Inalfa Part Number":string, "Serial Number":string, "Scanner Data 2":string, "Scanner Data 1 Ok":bool, "Scanner Data 2 Ok":bool}
  T49 = typedef "WKLXF25 St 60 PLC Data Control.ctl" = cluster{"Serial Number":string, "Inalfa Part Number":string, "Sunshade Color":string, "Shade 1 Barcode":string, "Shade 2 Barcode":string, "Model Type":string, "Part History Number":string, "Customer Number":string}
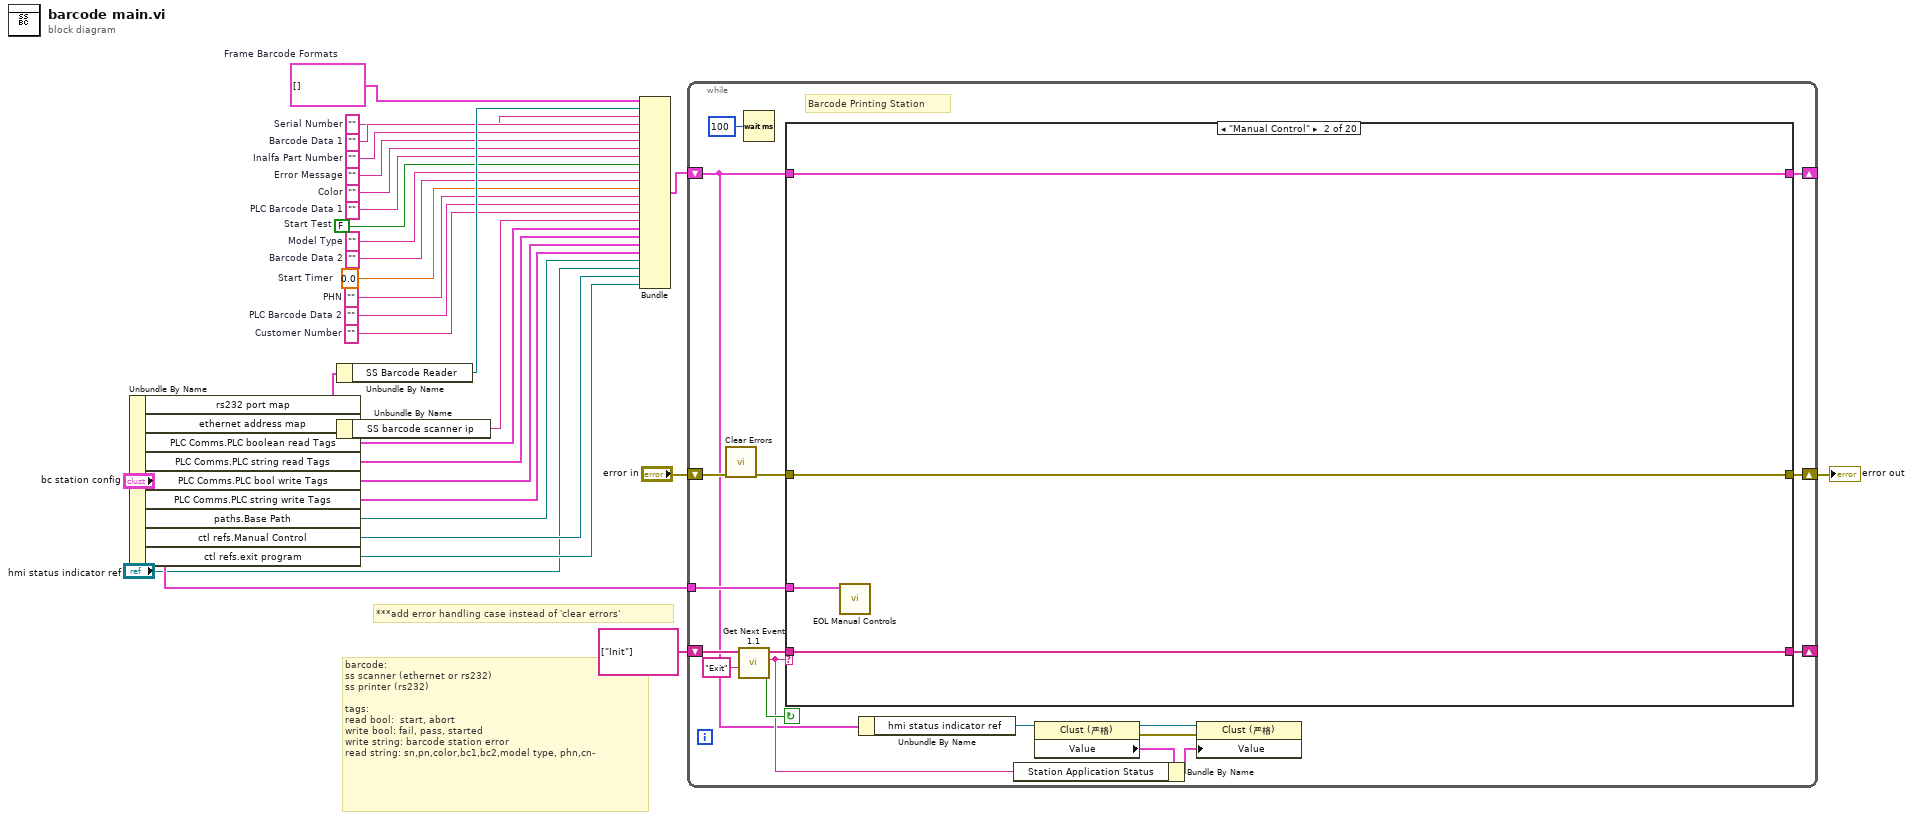
[diagram p0: block diagram]
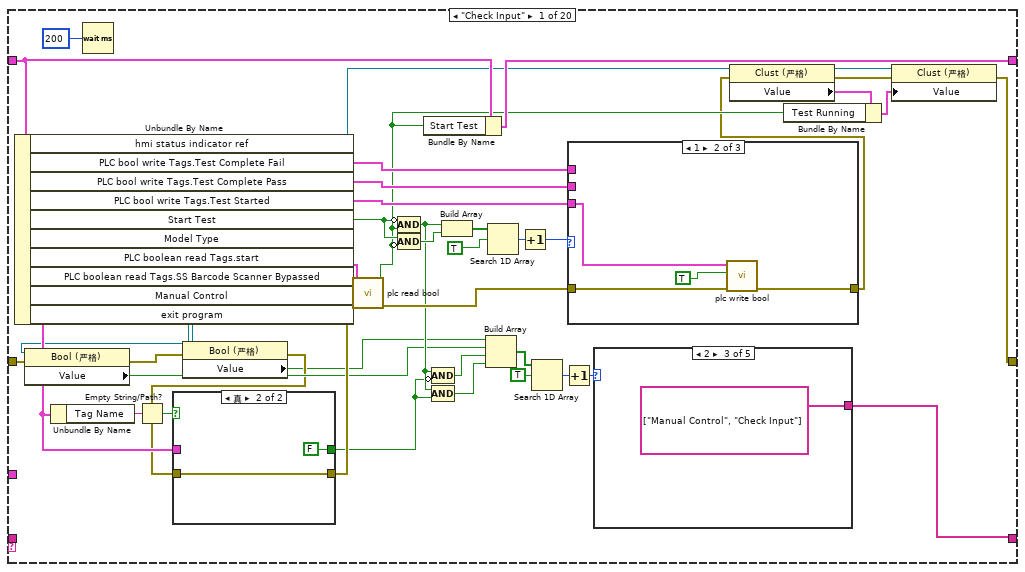
[diagram p2: hidden frame]
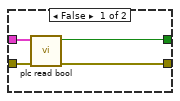
[diagram p3: hidden frame]
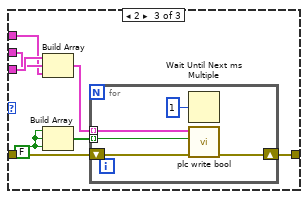
[diagram p5: hidden frame]
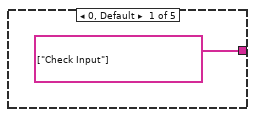
[diagram p6: hidden frame]
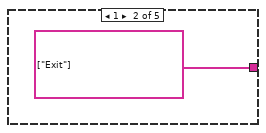
[diagram p7: hidden frame]
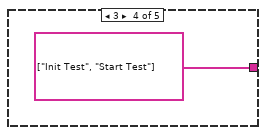
[diagram p8: hidden frame]
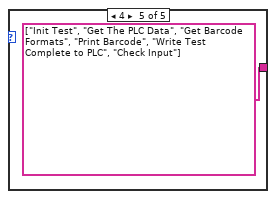
[diagram p9: hidden frame]
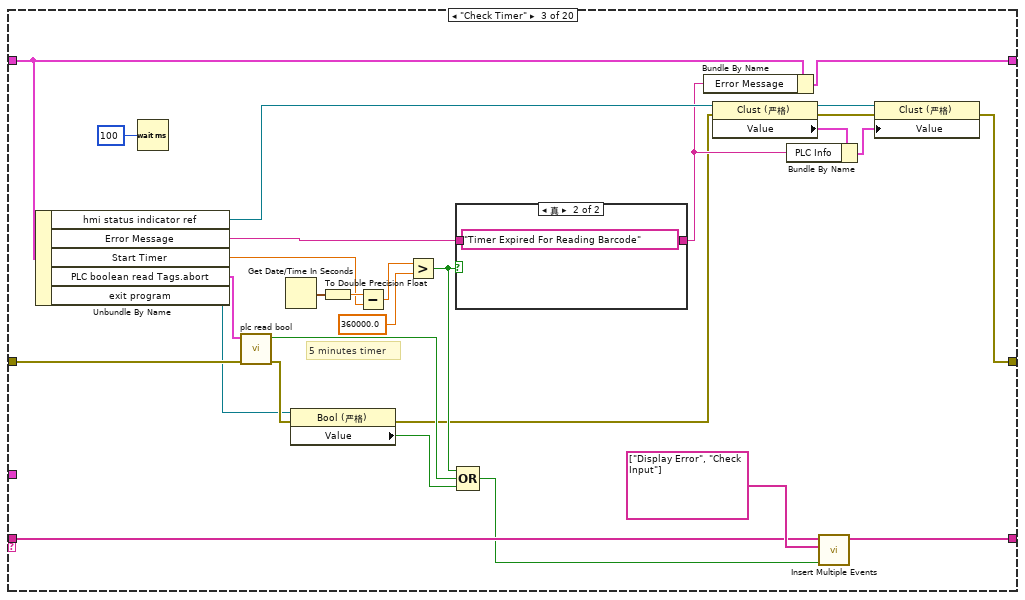
[diagram p10: hidden frame]
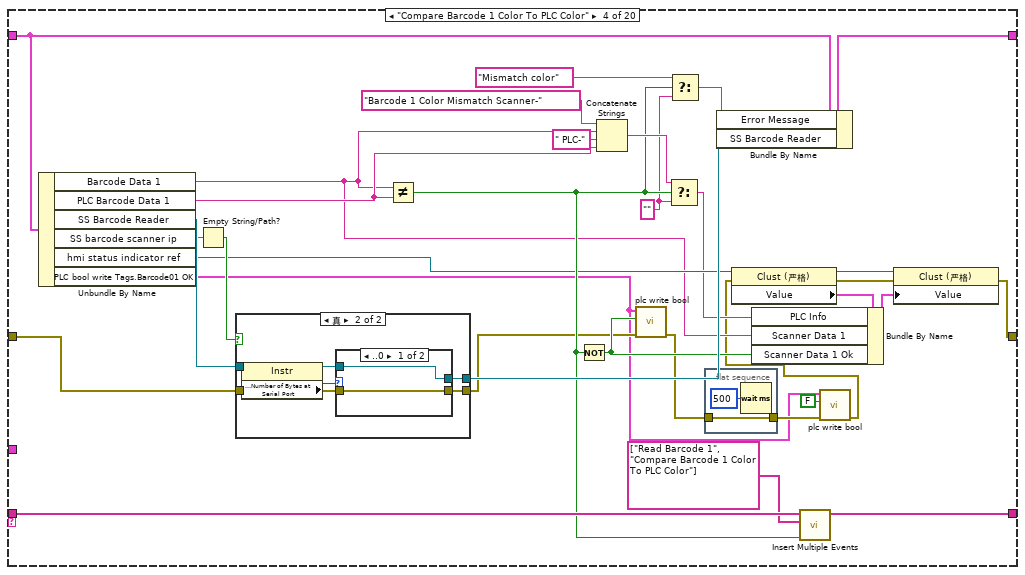
[diagram p12: hidden frame]
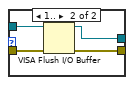
[diagram p14: hidden frame]
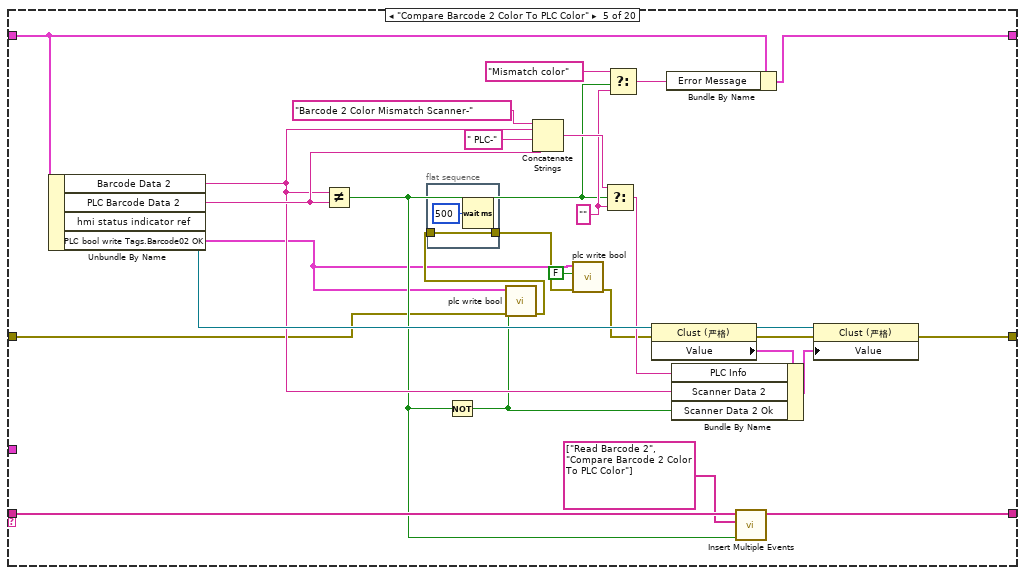
[diagram p15: hidden frame]
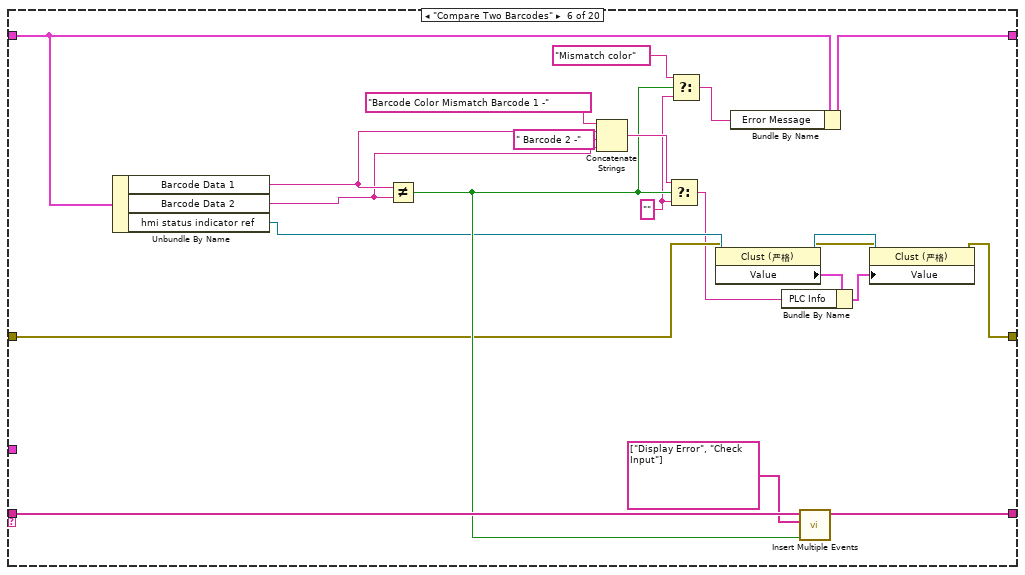
[diagram p16: hidden frame]
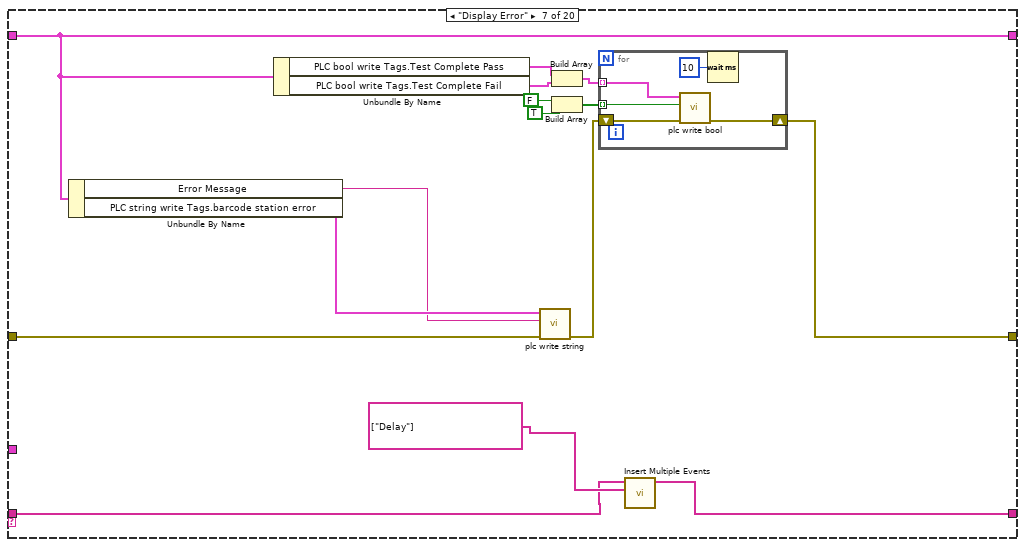
[diagram p17: hidden frame]
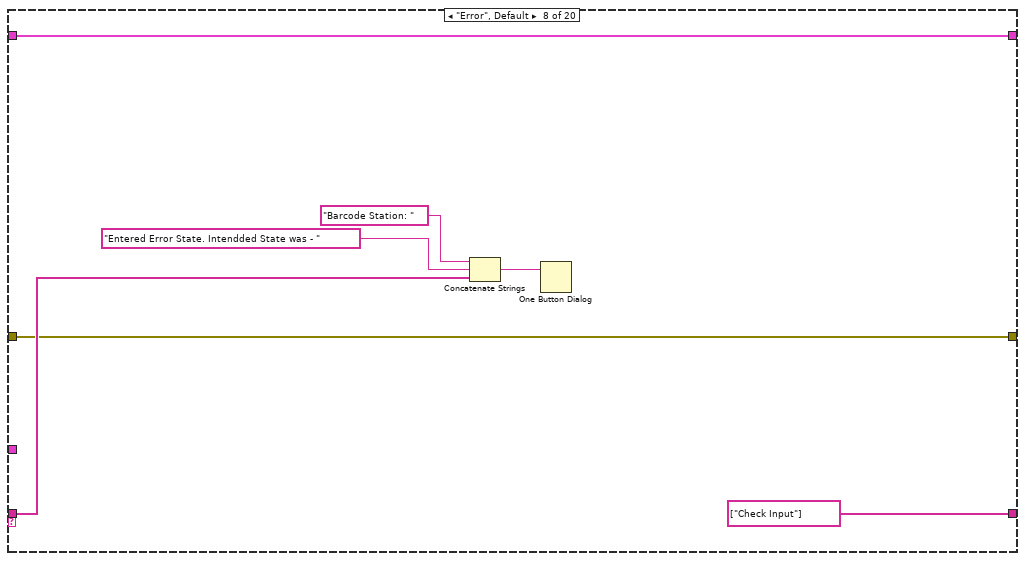
[diagram p18: hidden frame]
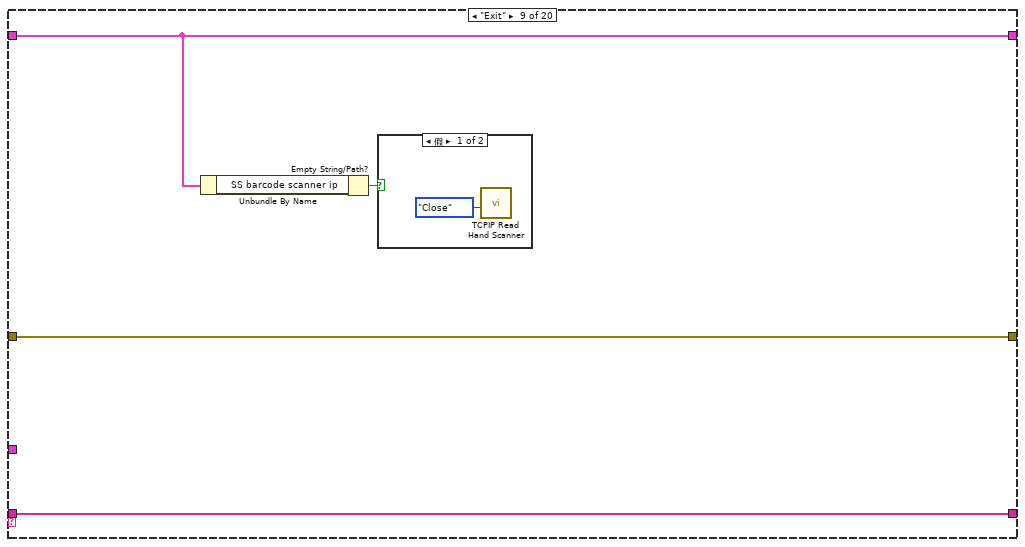
[diagram p19: hidden frame]
diagram:
  w27 = T45[] []  # Frame Barcode Formats
  w17 = ""  # Customer Number
  w16 = ""  # PLC Barcode Data 2
  w15 = ""  # PHN
  w14 = 0.0  # Start Timer
  w13 = ""  # Barcode Data 2
  w12 = ""  # Model Type
  w11 = FALSE  # Start Test
  w10 = ""  # PLC Barcode Data 1
  w9 = ""  # Color
  w8 = ""  # Error Message
  w7 = ""  # Inalfa Part Number
  w6 = ""  # Barcode Data 1
  w5 = ""  # Serial Number
  # "***add error handling case instead of 'clear errors'"
  # "barcode: \nss scanner (ethernet or rs232)\nss printer (rs232)\n\ntags:\nread bool:  start, abort\nwrite bool: fail, pass, started\nwrite string: barcode station error\nread string: sn,pn,color,bc1,bc2,model type, phn,cn-"
  n1 = Unbundle By Name("bc station config") -> ("rs232 port map"=w20:T9, "ethernet address map"=w18:T10, "PLC Comms.PLC boolean read Tags"=w22:T24, "PLC Comms.PLC string read Tags"=w23:T28, "PLC Comms.PLC bool write Tags"=w24:T27, "PLC Comms.PLC string write Tags"=w25:T29, "paths.Base Path"=w26:path, "ctl refs.Manual Control"=w31:refnum<vi>, "ctl refs.exit program"=w30:refnum<vi>)
  n2 = Unbundle By Name(w20) -> ("SS Barcode Reader"=w21:refnum<visa-resource-name>)
  n3 = Unbundle By Name(w18) -> ("SS barcode scanner ip"=w19:string)
  n4 = Bundle("Frame Barcode Formats"=w27, "SS Barcode Reader"=w21, "Serial Number"=w5, "Barcode Data 1"=w6, "Inalfa Part Number"=w7, "Error Message"=w8, "Color"=w9, "PLC Barcode Data 1"=w10, "Start Test"=w11, "Model Type"=w12, "Barcode Data 2"=w13, "Start Timer"=w14, "PHN"=w15, "PLC Barcode Data 2"=w16, "Customer Number"=w17, "SS barcode scanner ip"=w19, "PLC boolean read Tags"=w22, "PLC string read Tags"=w23, "PLC bool write Tags"=w24, "PLC string write Tags"=w25, "Base Path"=w26, "hmi status indicator ref"="hmi status indicator ref", "Manual Control"=w31, "exit program"=w30) -> (w4:T47)  [unwired: 1 in]
  n5 = while {
    shift-right: [w46] -> _
    shift-left: string[] ["Init"] ("event queue out") -> [w45]
    shift-right: [w44] -> _
    shift-left: w4 -> [w32]
    shift-right: [w42] -> w1
    shift-left: "error in" -> [w41]
    tunnel: "bc station config" -> [w39]
    stop <- w48 continue-if-true
    # "Barcode Printing Station"
    n6 = call <vilib>:"Clear Errors.vi"("error in (no error)"=w41) -> ("error out"=w40:errorcluster)  [unwired: 5 in, 1 out]
    n7 = call "Get Next Event 1.1.vi"("Exit Event"="Exit", "event queue in"=w45) -> ("Condition (Exit:F)"=w48:bool, "next event"=w33:string, "event queue out"=w47:string[])  [unwired: 6 in, 1 out]
    n8 = Wait (ms)(milliseconds to wait=u32 100) -> ()  [unwired: 1 out]
    n9 = case shown="\"Manual Control\"" w33 {
      tunnel: w47 -> [_ w124 w149 w186 w230 w254 w258 w279 w287 w310 _ w372 w390 w393 w412 w426 w482 w529 _ w565]
      tunnel: [w50 w124 w148 w187 w231 w255 w257 string[] ["Check Input"] ("event queue out") w287 w311 string[] ["Check Input"] ("event queue out") w372 w390 w392 w412 w427 w487 w529 w545 w565] -> w46
      tunnel: w32 -> [w85 w123 w151 w184 w228 w252 w261 w278 w286 w305 w327 w365 w389 w400 w413 w431 w486 w526 w544 w552]
      tunnel: [w84 w123 w147 w183 w227 w251 w261 w278 w286 w312 w326 w364 w389 w400 w413 w430 w485 w525 w544 w552] -> w44
      tunnel: [w58 w122 w130 w164 w214 w236 w262 w276 w283 w298 w316 w361 w382 w399 w414 w416 w472 w524 w532 w555] -> w42
      tunnel: w40 -> [w57 w122 w137 w176 w209 w237 w263 w276 w283 w299 w314 w362 w379 w395 w414 w417 w473 w524 w542 w561]
      tunnel: w39 -> [_ w121 _ _ _ _ _ _ _ _ _ _ _ _ _ _ _ _ _ _]
      frame "Check Input" {
        n10 = Unbundle By Name(w85) -> ("hmi status indicator ref"=w60:refnum<vi>, "PLC bool write Tags.Test Complete Fail"=w75:T25, "PLC bool write Tags.Test Complete Pass"=w76:T25, "PLC bool write Tags.Test Started"=w77:T25, "Start Test"=w90:bool, "PLC boolean read Tags.start"=w78:T25, "PLC boolean read Tags.SS Barcode Scanner Bypassed"=w71:T25, "Manual Control"=w56:refnum<vi>, "exit program"=w51:refnum<vi>)  [unwired: 1 out]
        n11 = property class="Bool (严格)"(reference=w56, error in=w57) -> (error out=w54:errorcluster, "Value"=w55:bool)  [unwired: 1 out]
        n12 = Unbundle By Name(w71) -> ("Tag Name"=w73:string)
        n13 = Wait (ms)(milliseconds to wait=u32 200) -> ()  [unwired: 1 out]
        n14 = Empty String/Path?(string/path=w73) -> (empty?=w72:bool)
        n15 = property class="Bool (严格)"(reference=w51, error in=w54) -> (error out=w53:errorcluster, "Value"=w52:bool)  [unwired: 1 out]
        n16 = case shown="真" w72 {
          tunnel: w53 -> [w95 w97]
          tunnel: w71 -> [w94 _]
          tunnel: [w93 w97] -> w70
          tunnel: [w92 FALSE ("value")] -> w67
          frame False {
            n17 = call "plc read bool.vi"("error in"=w95, "addr,tag"=w94) -> ("error out"=w93:errorcluster, "value"=w92:bool)  [unwired: 8 in]
          }
          frame True {
          }
        }
        n18 = call "plc read bool.vi"("error in"=w70, "addr,tag"=w78) -> ("error out"=w74:errorcluster, "value"=w61:bool)  [unwired: 8 in]
        n19 = Compound Arithmetic op=AND(invert w90, w61) -> (w68:bool)
        n20 = Compound Arithmetic op=AND(w90, invert w61) -> (w89:bool)
        n21 = Bundle By Name(cluster=w85, "Start Test"=w61) -> (w84:T47)
        n22 = Compound Arithmetic op=AND(w68, invert w67) -> (w69:bool)
        n23 = Compound Arithmetic op=AND(w68, w67) -> (w66:bool)
        n24 = Build Array(w68, w89) -> (w87:bool[])
        n25 = Build Array(w52, w55, w69, w66) -> (w81:bool[])
        n26 = Search 1D Array(1D array=w87, element=TRUE) -> (index of element=w88:i32)  [unwired: 1 in]
        n27 = Increment(x=w88) -> (x+1=w83:i32)
        n28 = Search 1D Array(1D array=w81, element=TRUE) -> (index of element=w80:i32)  [unwired: 1 in]
        n29 = Increment(x=w80) -> (x+1=w79:i32)
        n30 = case shown="1" w83 {
          tunnel: w77 -> [_ w102 w107]
          tunnel: w76 -> [_ _ w106]
          tunnel: w75 -> [_ _ w105]
          tunnel: w74 -> [w98 w100 w104]
          tunnel: [w98 w99 w103] -> w59
          frame 0, Default {
          }
          frame 1 {
            n31 = call "plc write bool.vi"("error in"=w100, "value"=TRUE, "addr,tag"=w102) -> ("error out"=w99:errorcluster)  [unwired: 8 in]
          }
          frame 2 {
            w108 = FALSE
            n32 = Build Array(w107, w106, w105) -> (w110:T25[])
            n33 = Build Array(w108, w108, w108) -> (w109:bool[])
            n34 = for {
              tunnel: w110 -> [w115] mode=indexing
              tunnel: w109 -> [w114] mode=indexing
              shift-right: [w112] -> w103
              shift-left: w104 -> [w113]
              n35 = Wait Until Next ms Multiple(millisecond multiple=u32 1) -> ()  [unwired: 1 out]
              n36 = call "plc write bool.vi"("error in"=w113, "value"=w114, "addr,tag"=w115) -> ("error out"=w112:errorcluster)  [unwired: 8 in]
            }
          }
        }
        n37 = case shown="2" w79 {
          tunnel: [string[] ["Check Input"] ("event queue out") string[] ["Exit"] ("event queue out") string[] ["Manual Control", "Check Input"] ("event queue out") string[] ["Init Test", "Start Test"] ("event queue out") string[] ["Init Test", "Get The PLC Data", "Get Barcode Formats", "Print Barcode", "Write Test Complete to PLC", "Check Input"] ("event queue out")] -> w50
          frame 0, Default {
          }
          frame 1 {
          }
          frame 2 {
          }
          frame 3 {
          }
          frame 4 {
          }
        }
        n38 = property class="Clust (严格)"(reference=w60, error in=w59) -> (reference out=w65:refnum<vi>, error out=w63:errorcluster, "Value"=w64:T48)
        n39 = Bundle By Name(cluster=w64, "Test Running"=w61) -> (w62:T48)
        n40 = property class="Clust (严格)"(reference=w65, error in=w63, "Value"=w62) -> (error out=w58:errorcluster)  [unwired: 1 out]
      }
      frame "Manual Control" {
        n41 = call "EOL Manual Controls.vi"("main thread cluster"=w121) -> ()  [unwired: 10 in, 1 out]
      }
      frame "Check Timer" {
        # "5 minutes timer"
        n42 = Unbundle By Name(w151) -> ("hmi status indicator ref"=w131:refnum<vi>, "Error Message"=w146:string, "Start Timer"=w143:dbl, "PLC boolean read Tags.abort"=w138:T25, "exit program"=w126:refnum<vi>)
        n43 = Wait (ms)(milliseconds to wait=u32 100) -> ()  [unwired: 1 out]
        n44 = call "plc read bool.vi"("error in"=w137, "addr,tag"=w138) -> ("error out"=w128:errorcluster, "value"=w136:bool)  [unwired: 8 in]
        n45 = Get Date/Time In Seconds() -> (seconds since 1Jan1904=w145:timestamp)
        n46 = property class="Bool (严格)"(reference=w126, error in=w128) -> (error out=w127:errorcluster, "Value"=w125:bool)  [unwired: 1 out]
        n47 = To Double Precision Float(number=w145) -> (double precision float=w144:dbl)
        n48 = Subtract(x=w144, y=w143) -> (x-y=w142:dbl)
        n49 = Greater?(x=w142, y=360000.0) -> (0:w141:bool)
        n50 = case shown="真" w141 {
          tunnel: w146 -> [w153 _]
          tunnel: [w153 "Timer Expired For Reading Barcode" ("Error Message")] -> w129
          frame False {
          }
          frame True {
          }
        }
        n51 = Compound Arithmetic op=OR(w141, w136, w125) -> (w140:bool)
        n52 = Bundle By Name(cluster=w151, "Error Message"=w129) -> (w147:T47)
        n53 = property class="Clust (严格)"(reference=w131, error in=w127) -> (reference out=w132:refnum<vi>, error out=w133:errorcluster, "Value"=w134:T48)
        n54 = Bundle By Name(cluster=w134, "PLC Info"=w129) -> (w135:T48)
        n55 = call "Insert Multiple Events.vi"("Insert all? (T)"=w140, "Events to Insert"=string[] ["Display Error", "Check Input"] ("f"), "Event queue in"=w149) -> ("Event queue out"=w148:string[])  [unwired: 4 in]
        n56 = property class="Clust (严格)"(reference=w132, error in=w133, "Value"=w135) -> (error out=w130:errorcluster)  [unwired: 1 out]
      }
      frame "Compare Barcode 1 Color To PLC Color" {
        w173 = ""
        n57 = Unbundle By Name(w184) -> ("Barcode Data 1"=w162:string, "PLC Barcode Data 1"=w179:string, "SS Barcode Reader"=w178:refnum<visa-resource-name>, "SS barcode scanner ip"=w171:string, "hmi status indicator ref"=w165:refnum<vi>, "PLC bool write Tags.Barcode01 OK"=w157:T25)
        n58 = Empty String/Path?(string/path=w171) -> (empty?=w170:bool)
        n59 = case shown="真" w170 {
          tunnel: w178 -> [w191 w197]
          tunnel: [w191 w196] -> w177
          tunnel: w176 -> [w190 w193]
          tunnel: [w190 w192] -> w160
          frame False {
          }
          frame True {
            n60 = property class="Instr"(reference=w197) -> (reference out=w194:refnum<visa-resource-name>, "Serial Settings:Number of Bytes at Serial Port"=w195:u32)  [unwired: 1 in, 1 out]
            n61 = case shown="..0" w195 {
              tunnel: [w199 w203] -> w196
              tunnel: w194 -> [w199 w202]
              tunnel: w193 -> [w198 w201]
              tunnel: [w198 w200] -> w192
              frame ..0 {
              }
              frame 1.. {
                n62 = VISA Flush I/O Buffer(VISA resource name=w202, error in (no error)=w201) -> (VISA resource name out=w203:refnum<visa-resource-name>, error out=w200:errorcluster)  [unwired: 1 in]
              }
            }
          }
        }
        n63 = Not Equal?(x=w162, y=w179) -> (x != y?=w174:bool)
        n64 = Not(x=w174) -> (.not. x?=w161:bool)
        n65 = Concatenate Strings("Barcode 1 Color Mismatch Scanner-" ("t"), w162, " PLC-" ("string"), w179) -> (w182:string)
        n66 = call "plc write bool.vi"("error in"=w160, "value"=w161, "addr,tag"=w157) -> ("error out"=w159:errorcluster)  [unwired: 8 in]
        n67 = Select(t=w182, s=w174, f=w173) -> (s? t:f=w163:string)
        n68 = Select(t="Mismatch color", s=w174, f=w173) -> (s? t:f=w172:string)
        n69 = flat-sequence {
          tunnel: w159 -> [w188]
          tunnel: [w188] -> w158
          frame #0 {
            n70 = Wait (ms)(milliseconds to wait=u32 500) -> ()  [unwired: 1 out]
          }
        }
        n71 = Bundle By Name(cluster=w184, "Error Message"=w172, "SS Barcode Reader"=w177) -> (w183:T47)
        n72 = call "Insert Multiple Events.vi"("Insert all? (T)"=w174, "Events to Insert"=string[] ["Read Barcode 1", "Compare Barcode 1 Color To PLC Color"], "Event queue in"=w186) -> ("Event queue out"=w187:string[])  [unwired: 4 in]
        n73 = call "plc write bool.vi"("error in"=w158, "value"=FALSE, "addr,tag"=w157) -> ("error out"=w155:errorcluster)  [unwired: 8 in]
        n74 = property class="Clust (严格)"(reference=w165, error in=w155) -> (reference out=w166:refnum<vi>, error out=w167:errorcluster, "Value"=w168:T48)
        n75 = Bundle By Name(cluster=w168, "PLC Info"=w163, "Scanner Data 1"=w162, "Scanner Data 1 Ok"=w161) -> (w169:T48)
        n76 = property class="Clust (严格)"(reference=w166, error in=w167, "Value"=w169) -> (error out=w164:errorcluster)  [unwired: 1 out]
      }
      frame "Compare Barcode 2 Color To PLC Color" {
        w221 = ""
        n77 = Unbundle By Name(w228) -> ("Barcode Data 2"=w212:string, "PLC Barcode Data 2"=w223:string, "hmi status indicator ref"=w215:refnum<vi>, "PLC bool write Tags.Barcode02 OK"=w208:T25)
        n78 = Not Equal?(x=w212, y=w223) -> (x != y?=w210:bool)
        n79 = flat-sequence {
          tunnel: w211 -> [w232]
          tunnel: [w232] -> w207
          frame #0 {
            n80 = Wait (ms)(milliseconds to wait=u32 500) -> ()  [unwired: 1 out]
          }
        }
        n81 = Not(x=w210) -> (.not. x?=w204:bool)
        n82 = call "plc write bool.vi"("error in"=w209, "value"=w204, "addr,tag"=w208) -> ("error out"=w211:errorcluster)  [unwired: 8 in]
        n83 = Concatenate Strings("Barcode 2 Color Mismatch Scanner-" ("t"), w212, " PLC-" ("string"), w223) -> (w226:string)
        n84 = call "plc write bool.vi"("error in"=w207, "value"=FALSE, "addr,tag"=w208) -> ("error out"=w206:errorcluster)  [unwired: 8 in]
        n85 = Select(t=w226, s=w210, f=w221) -> (s? t:f=w213:string)
        n86 = Select(t="Mismatch color", s=w210, f=w221) -> (s? t:f=w220:string)
        n87 = property class="Clust (严格)"(reference=w215, error in=w206) -> (reference out=w219:refnum<vi>, error out=w216:errorcluster, "Value"=w217:T48)
        n88 = Bundle By Name(cluster=w228, "Error Message"=w220) -> (w227:T47)
        n89 = Bundle By Name(cluster=w217, "PLC Info"=w213, "Scanner Data 2"=w212, "Scanner Data 2 Ok"=w204) -> (w218:T48)
        n90 = call "Insert Multiple Events.vi"("Insert all? (T)"=w210, "Events to Insert"=string[] ["Read Barcode 2", "Compare Barcode 2 Color To PLC Color"], "Event queue in"=w230) -> ("Event queue out"=w231:string[])  [unwired: 4 in]
        n91 = property class="Clust (严格)"(reference=w219, error in=w216, "Value"=w218) -> (error out=w214:errorcluster)  [unwired: 1 out]
      }
      frame "Compare Two Barcodes" {
        w243 = ""
        n92 = Unbundle By Name(w252) -> ("Barcode Data 1"=w248:string, "Barcode Data 2"=w246:string, "hmi status indicator ref"=w238:refnum<vi>)
        n93 = Not Equal?(x=w248, y=w246) -> (x != y?=w245:bool)
        n94 = Concatenate Strings("Barcode Color Mismatch Barcode 1 -" ("t"), w248, " Barcode 2 -" ("string"), w246) -> (w250:string)
        n95 = Select(t=w250, s=w245, f=w243) -> (s? t:f=w234:string)
        n96 = Select(t="Mismatch color", s=w245, f=w243) -> (s? t:f=w242:string)
        n97 = property class="Clust (严格)"(reference=w238, error in=w237) -> (reference out=w241:refnum<vi>, error out=w239:errorcluster, "Value"=w240:T48)
        n98 = Bundle By Name(cluster=w252, "Error Message"=w242) -> (w251:T47)
        n99 = Bundle By Name(cluster=w240, "PLC Info"=w234) -> (w235:T48)
        n100 = call "Insert Multiple Events.vi"("Insert all? (T)"=w245, "Events to Insert"=string[] ["Display Error", "Check Input"], "Event queue in"=w254) -> ("Event queue out"=w255:string[])  [unwired: 4 in]
        n101 = property class="Clust (严格)"(reference=w241, error in=w239, "Value"=w235) -> (error out=w236:errorcluster)  [unwired: 1 out]
      }
      frame "Display Error" {
        n102 = Unbundle By Name(w261) -> ("Error Message"=w256:string, "PLC string write Tags.barcode station error"=w260:T25)
        n103 = Unbundle By Name(w261) -> ("PLC bool write Tags.Test Complete Pass"=w270:T25, "PLC bool write Tags.Test Complete Fail"=w269:T25)
        n104 = call "plc write string.vi"("error in"=w263, "value"=w256, "addr,tag"=w260) -> ("error out"=w264:errorcluster)  [unwired: 8 in]
        n105 = Build Array(w270, w269) -> (w268:T25[])
        n106 = Build Array(FALSE, TRUE ("element")) -> (w266:bool[])
        n107 = for {
          tunnel: w268 -> [w273] mode=indexing
          tunnel: w266 -> [w272] mode=indexing
          shift-right: [w274] -> w262
          shift-left: w264 -> [w275]
          n108 = call "plc write bool.vi"("error in"=w275, "value"=w272, "addr,tag"=w273) -> ("error out"=w274:errorcluster)  [unwired: 8 in]
          n109 = Wait (ms)(milliseconds to wait=u32 10) -> ()  [unwired: 1 out]
        }
        n110 = call "Insert Multiple Events.vi"("Events to Insert"=string[] ["Delay"] ("event queue out"), "Event queue in"=w258) -> ("Event queue out"=w257:string[])  [unwired: 5 in]
      }
      frame "Error", Default {
        n111 = Concatenate Strings("Barcode Station: " ("string"), "Entered Error State. Intendded State was - " ("string"), w279) -> (w282:string)
        n112 = One Button Dialog(message=w282) -> ()  [unwired: 1 in, 1 out]
      }
      frame "Exit" {
        n113 = Unbundle By Name(w286) -> ("SS barcode scanner ip"=w284:string)
        n114 = Empty String/Path?(string/path=w284) -> (empty?=w285:bool)
        n115 = case shown="假" w285 {
          frame False {
            n116 = call "TCPIP Read Hand Scanner.vi"("Mode"=enum16{"Init", "Read", "Close"}."Close") -> ()  [unwired: 10 in, 1 out]
          }
          frame True {
          }
        }
      }
      frame "Get The PLC Data" {
        n117 = Unbundle By Name(w305) -> ("PLC string read Tags"=w304:T28, "hmi status indicator ref"=w289:refnum<vi>)
        n118 = call "WKLXF25 St 60 PLC Data 2.0.vi"("PLC string read Tags"=w304) -> ("No Data?"=w306:bool, "Error String"=w307:string, "PLC Data"=w308:T49)  [unwired: 6 in]
        n119 = Unbundle By Name(w308) -> ("Serial Number"=w297:string, "Inalfa Part Number"=w296:string, "Sunshade Color"=w295:string, "Shade 1 Barcode"=w294:string, "Shade 2 Barcode"=w293:string, "Model Type"=w292:string, "Part History Number"=w291:string, "Customer Number"=w290:string)
        n120 = call "Insert Multiple Events.vi"("Insert all? (T)"=w306, "Events to Insert"=string[] ["Display Error", "Check Input"], "Event queue in"=w310) -> ("Event queue out"=w311:string[])  [unwired: 4 in]
        n121 = property class="Clust (严格)"(reference=w289, error in=w299) -> (reference out=w303:refnum<vi>, error out=w301:errorcluster, "Value"=w302:T48)
        n122 = Bundle By Name(cluster=w302, "Serial Number"=w297, "Inalfa Part Number"=w296, "Color"=w295, "PLC Barcode Data 1"=w294, "PLC Barcode Data 2"=w293, "Model Type"=w292, "PHN"=w291, "Customer Number"=w290) -> (w300:T48)
        n123 = Bundle By Name(cluster=w305, "Serial Number"=w297, "Inalfa Part Number"=w296, "Color"=w295, "PLC Barcode Data 1"=w294, "PLC Barcode Data 2"=w293, "Model Type"=w292, "PHN"=w291, "Customer Number"=w290, "Error Message"=w307) -> (w312:T47)
        n124 = property class="Clust (严格)"(reference=w303, error in=w301, "Value"=w300) -> (error out=w298:errorcluster)  [unwired: 1 out]
      }
      frame "Init" {
        n125 = Unbundle By Name(w327) -> ("SS Barcode Reader"=w325:refnum<visa-resource-name>, "SS barcode scanner ip"=w322:string, "PLC bool write Tags"=w321:T27)  [unwired: 3 out]
        n126 = Empty String/Path?(string/path=w322) -> (empty?=w323:bool)
        n127 = Unbundle By Name(w321) -> ("Test Complete Pass"=w320:T25, "Test Complete Fail"=w319:T25, "Test Started"=w318:T25)
        n128 = case shown="真" w323 {
          tunnel: w325 -> [w338 w345]
          tunnel: [w338 w342] -> w324
          tunnel: w322 -> [w335 _]
          tunnel: w314 -> [w334 w341]
          tunnel: [w334 w339] -> w315
          frame False {
            n129 = call "TCPIP Read Hand Scanner.vi"("Mode"=enum16{"Init", "Read", "Close"}."Init", "remote port or service name"=u16 9004, "address"=w335) -> ()  [unwired: 8 in, 1 out]
          }
          frame True {
            w343 = u16 0 items=["None"=0, "XON/XOFF"=1, "RTS/CTS"=2, "DTR/DSR"=4] ("flow control")
            w344 = u16 10 items=["1.0"=10, "1.5"=15, "2.0"=20] ("stop bits")
            w347 = u16 2 items=["None", "Odd", "Even", "Mark", "Space"] ("parity")
            w349 = FALSE  # Enable Termination Char (T)
            w348 = u32 10000  # timeout (10sec)
            n130 = call-poly "VISA Configure Serial Port"("VISA resource name"=w345, "timeout (10sec)"=w348, "Enable Termination\nChar (T)"=w349, "baud rate (9600)"=u32 9600 ("baud rate"), "data bits (8)"=u16 7 ("data bits"), "parity (0:none)"=w347, "error in (no error)"=w341, "stop bits (10: 1 bit)"=w344, "flow control (0:none)"=w343) -> ("VISA resource name out"=w353:refnum<visa-resource-name>, "error out"=w354:errorcluster)  [unwired: 5 in]
            n131 = property class="Instr"(reference=w353, error in=w354) -> (reference out=w351:refnum<visa-resource-name>, error out=w340:errorcluster, "Serial Settings:Number of Bytes at Serial Port"=w352:u32)
            n132 = case shown="1.." w352 {
              tunnel: [w356 w360] -> w342
              tunnel: w351 -> [w356 w359]
              tunnel: w340 -> [w355 w358]
              tunnel: [w355 w357] -> w339
              frame ..0 {
              }
              frame 1.. {
                n133 = VISA Flush I/O Buffer(VISA resource name=w359, error in (no error)=w358) -> (VISA resource name out=w360:refnum<visa-resource-name>, error out=w357:errorcluster)  [unwired: 1 in]
              }
            }
          }
        }
        n134 = Build Array(w320, w319, w318) -> (w317:T25[])
        n135 = Bundle By Name(cluster=w327, "SS Barcode Reader"=w324) -> (w326:T47)
        n136 = for {
          tunnel: w317 -> [w333] mode=indexing
          shift-right: [w331] -> w316
          shift-left: w315 -> [w332]
          tunnel: bool[] [FALSE, FALSE, TRUE] -> [w329] mode=indexing
          n137 = call "plc write bool.vi"("error in"=w332, "value"=w329, "addr,tag"=w333) -> ("error out"=w331:errorcluster)  [unwired: 8 in]
          n138 = Wait (ms)(milliseconds to wait=u32 10) -> ()  [unwired: 1 out]
        }
      }
      frame "Get Barcode Formats" {
        n139 = Unbundle By Name(w365) -> ("Base Path"=w371:path, "Model Type"=w369:string)
        n140 = call "get path to barcode formats.vi"("product"=w369, "paths.Base Path"=w371) -> ("path"=w370:path)  [unwired: 9 in]
        n141 = call <vilib>:"Check if File or Folder Exists.vi"("error in (no error)"=w362, "path"=w370) -> ("error out"=w366:errorcluster, "file or folder exists?"=w368:bool, "dup path"=w367:path)  [unwired: 7 in]
        n142 = case shown="真" w368 {
          tunnel: w367 -> [_ w378]
          tunnel: w366 -> [w374 w377]
          tunnel: [w374 w376] -> w361
          tunnel: [T45[] [] ("Frame Barcode Formats") w375] -> w363
          frame False {
          }
          frame True {
            n143 = call "read barcode formats.vi"("error in"=w377, "configuration file path"=w378) -> ("error out"=w376:errorcluster, "Frame Barcode Formats"=w375:T45[])  [unwired: 8 in]
          }
        }
        n144 = Bundle By Name(cluster=w365, "Frame Barcode Formats"=w363) -> (w364:T47)
      }
      frame "Print Barcode" {
        n145 = Unbundle By Name(w389) -> ("Inalfa Part Number"=w385:string, "Serial Number"=w384:string, "Color"=w380:string, "PHN"=w386:string, "Customer Number"=w381:string, "Frame Barcode Formats"=w388:T45[], "Model Type"=w383:string)
        n146 = call "Barcode Print.vi"("part type"=w383, "Manual?"=FALSE, "error in"=w379, "Part History Number"=w386, "Customer Number"=w381, "Color"=w380, "Serial Number"=w384, "Inalfa Part Number"=w385, "Frame Barcode Formats"=w388) -> ("error out"=w382:errorcluster)  [unwired: 2 in]
      }
      frame "Write Test Complete to PLC" {
        n147 = Unbundle By Name(w400) -> ("PLC bool write Tags.Test Complete Pass"=w406:T25, "PLC bool write Tags.Test Complete Fail"=w405:T25, "PLC string write Tags.barcode station error"=w398:T25)
        n148 = call "plc write string.vi"("error in"=w395, "value"="Barcode Printed OK", "addr,tag"=w398) -> ("error out"=w397:errorcluster)  [unwired: 8 in]
        n149 = call "Insert Multiple Events.vi"("Events to Insert"=string[] ["Delay"] ("event queue out"), "Event queue in"=w393) -> ("Event queue out"=w392:string[])  [unwired: 5 in]
        n150 = call <vilib>:"Clear Errors.vi"("error in (no error)"=w397) -> ("error out"=w391:errorcluster)  [unwired: 5 in, 1 out]
        n151 = Build Array(w406, w405) -> (w404:T25[])
        n152 = Build Array(TRUE, FALSE ("element")) -> (w402:bool[])
        n153 = for {
          tunnel: w404 -> [w411] mode=indexing
          tunnel: w402 -> [w410] mode=indexing
          shift-right: [w408] -> w399
          shift-left: w391 -> [w409]
          n154 = call "plc write bool.vi"("error in"=w409, "value"=w410, "addr,tag"=w411) -> ("error out"=w408:errorcluster)  [unwired: 8 in]
          n155 = Wait (ms)(milliseconds to wait=u32 10) -> ()  [unwired: 1 out]
        }
      }
      frame "Delay" {
        n156 = Wait (ms)(milliseconds to wait=u32 100) -> ()  [unwired: 1 out]
      }
      frame "Read Barcode 1" {
        n157 = Unbundle By Name(w431) -> ("Model Type"=w424:string, "SS Barcode Reader"=w418:refnum<visa-resource-name>, "SS barcode scanner ip"=w420:string)
        n158 = Empty String/Path?(string/path=w420) -> (empty?=w419:bool)
        n159 = case shown="真" w419 {
          tunnel: [w433 w438] -> w422
          tunnel: w418 -> [_ w440]
          tunnel: w417 -> [w432 w437]
          tunnel: [w432 w435] -> w416
          frame False {
            n160 = call "TCPIP Read Hand Scanner.vi"("Mode"=enum16{"Init", "Read", "Close"}."Read") -> ("String"=w433:string)  [unwired: 10 in]
          }
          frame True {
            n161 = property class="Instr"(reference=w440, error in=w437) -> (error out=w436:errorcluster, "Serial Settings:Number of Bytes at Serial Port"=w439:u32)  [unwired: 1 out]
            n162 = VISA Read(VISA resource name=w440, byte count=w439, error in (no error)=w436) -> (read buffer=w438:string, error out=w435:errorcluster)  [unwired: 2 out]
          }
        }
        n163 = To Upper Case(1:w422) -> (0:w421:string)
        n164 = Empty String/Path?(string/path=w421) -> (empty?=w423:bool)
        n165 = case shown="\"GMT166\"" w424 {
          tunnel: w421 -> [w442 w445 w448 w451 w454 w459 w464 w468 w470]
          tunnel: [w441 w444 w447 w450 w453 w457 w462 w467 w469] -> w425
          frame "WK", Default {
            n166 = String Subset(string=w442, length (rest)=3 ("length (rest)")) -> (substring=w441:string)  [unwired: 1 in]
          }
          frame "GMT166" {
            n167 = String Subset(string=w445, length (rest)=3 ("length (rest)")) -> (substring=w444:string)  [unwired: 1 in]
          }
          frame "LX" {
            n168 = String Subset(string=w448, length (rest)=3 ("length (rest)")) -> (substring=w447:string)  [unwired: 1 in]
          }
          frame "CD3" {
            n169 = String Subset(string=w451, length (rest)=8 ("length (rest)")) -> (substring=w450:string)  [unwired: 1 in]
          }
          frame "CD4" {
            n170 = String Subset(string=w454, length (rest)=8 ("length (rest)")) -> (substring=w453:string)  [unwired: 1 in]
          }
          frame "C520" {
            n171 = String Subset(string=w459, length (rest)=3 ("length (rest)")) -> (substring=w458:string)  [unwired: 1 in]
            n172 = Concatenate Strings("300217" ("string"), w458) -> (w457:string)
          }
          frame "CD391" {
            n173 = String Subset(string=w464, length (rest)=3 ("length (rest)")) -> (substring=w463:string)  [unwired: 1 in]
            n174 = Concatenate Strings("300217" ("string"), w463) -> (w462:string)
          }
          frame "F25" {
            n175 = Match Pattern(string=w468, regular expression="\r") -> (before substring=w467:string)  [unwired: 1 in, 3 out]
          }
          frame "F15" {
            n176 = Match Pattern(string=w470, regular expression="\r") -> (before substring=w469:string)  [unwired: 1 in, 3 out]
          }
        }
        n177 = Bundle By Name(cluster=w431, "Barcode Data 1"=w425, "Error Message"="" ("Inalfa Part Number")) -> (w430:T47)
        n178 = call "Insert Multiple Events.vi"("Insert all? (T)"=w423, "Events to Insert"=string[] ["Check Timer", "Read Barcode 1"] ("f"), "Event queue in"=w426) -> ("Event queue out"=w427:string[])  [unwired: 4 in]
      }
      frame "Read Barcode 2" {
        n179 = Unbundle By Name(w486) -> ("Model Type"=w479:string, "SS Barcode Reader"=w475:refnum<visa-resource-name>, "SS barcode scanner ip"=w474:string)
        n180 = Empty String/Path?(string/path=w474) -> (empty?=w477:bool)
        n181 = case shown="真" w477 {
          tunnel: [w489 w494] -> w476
          tunnel: w475 -> [_ w496]
          tunnel: w473 -> [w488 w493]
          tunnel: [w488 w491] -> w472
          frame False {
            n182 = call "TCPIP Read Hand Scanner.vi"("Mode"=enum16{"Init", "Read", "Close"}."Read") -> ("String"=w489:string)  [unwired: 10 in]
          }
          frame True {
            n183 = property class="Instr"(reference=w496, error in=w493) -> (error out=w492:errorcluster, "Serial Settings:Number of Bytes at Serial Port"=w495:u32)  [unwired: 1 out]
            n184 = VISA Read(VISA resource name=w496, byte count=w495, error in (no error)=w492) -> (read buffer=w494:string, error out=w491:errorcluster)  [unwired: 2 out]
          }
        }
        n185 = To Upper Case(1:w476) -> (0:w480:string)
        n186 = Empty String/Path?(string/path=w480) -> (empty?=w481:bool)
        n187 = case shown="\"WK\", 默认" w479 {
          tunnel: w480 -> [w498 w501 w504 w507 w510 w513 w516 w520 w522]
          tunnel: [w497 w500 w503 w506 w509 w512 w515 w519 w521] -> w478
          frame "WK", Default {
            n188 = String Subset(string=w498, length (rest)=3 ("length (rest)")) -> (substring=w497:string)  [unwired: 1 in]
          }
          frame "GMT166" {
            n189 = String Subset(string=w501, length (rest)=3 ("length (rest)")) -> (substring=w500:string)  [unwired: 1 in]
          }
          frame "LX" {
            n190 = String Subset(string=w504, length (rest)=3 ("length (rest)")) -> (substring=w503:string)  [unwired: 1 in]
          }
          frame "CD3" {
            n191 = String Subset(string=w507, length (rest)=8 ("length (rest)")) -> (substring=w506:string)  [unwired: 1 in]
          }
          frame "CD4" {
            n192 = String Subset(string=w510, length (rest)=8 ("length (rest)")) -> (substring=w509:string)  [unwired: 1 in]
          }
          frame "C520" {
            n193 = String Subset(string=w513, length (rest)=8 ("length (rest)")) -> (substring=w512:string)  [unwired: 1 in]
          }
          frame "CD391" {
            n194 = String Subset(string=w516, length (rest)=8 ("length (rest)")) -> (substring=w515:string)  [unwired: 1 in]
          }
          frame "F25" {
            n195 = Match Pattern(string=w520, regular expression="\r") -> (before substring=w519:string)  [unwired: 1 in, 3 out]
          }
          frame "F15" {
            n196 = Match Pattern(string=w522, regular expression="\r") -> (before substring=w521:string)  [unwired: 1 in, 3 out]
          }
        }
        n197 = Bundle By Name(cluster=w486, "Barcode Data 2"=w478, "Error Message"="" ("Inalfa Part Number")) -> (w485:T47)
        n198 = call "Insert Multiple Events.vi"("Insert all? (T)"=w481, "Events to Insert"=string[] ["Check Timer", "Read Barcode 2"] ("f"), "Event queue in"=w482) -> ("Event queue out"=w487:string[])  [unwired: 4 in]
      }
      frame "Set Timer" {
        n199 = Get Date/Time In Seconds() -> (seconds since 1Jan1904=w528:timestamp)
        n200 = To Double Precision Float(number=w528) -> (double precision float=w527:dbl)
        n201 = Bundle By Name(cluster=w526, "Start Timer"=w527) -> (w525:T47)
      }
      frame "Start Test" {
        # "Barcode Printing St Clear the Error message"
        n202 = Unbundle By Name(w544) -> ("hmi status indicator ref"=w530:refnum<vi>, "PLC string write Tags.barcode station error"=w539:T25, "PLC string read Tags.Model Type"=w543:T25)
        n203 = call "plc read string.vi"("error in"=w542, "addr,tag"=w543) -> ("error out"=w540:errorcluster, "Data"=w541:string)  [unwired: 8 in]
        n204 = case shown="默认" w541 {
          tunnel: [string[] ["Set Timer", "Get The PLC Data", "Get Barcode Formats", "Print Barcode", "Write Test Complete to PLC", "Check Input"] ("event queue out") string[] ["Set Timer", "Get The PLC Data", "Get Barcode Formats", "Print Barcode", "Write Test Complete to PLC", "Check Input"] ("event queue out") string[] ["Set Timer", "Get The PLC Data", "Get Barcode Formats", "Print Barcode", "Read Barcode 1", "Compare Barcode 1 Color To PLC Color", "Write Test Complete to PLC", "Check Input"] ("event queue out") string[] ["Set Timer", "Get The PLC Data", "Get Barcode Formats", "Read Barcode 1", "Compare Barcode 1 Color To PLC Color", "Print Barcode", "Set Timer", "Read Barcode 2", "Compare Barcode 2 Color To PLC Color", "Write Test Complete to PLC", "Check Input"] ("event queue out") string[] ["Set Timer", "Get The PLC Data", "Get Barcode Formats", "Print Barcode", "Read Barcode 1", "Compare Barcode 1 Color To PLC Color", "Write Test Complete to PLC", "Check Input"] ("event queue out")] -> w545
          frame Default {
          }
          frame "C53F", "CS11" {
          }
          frame "F15", "F25", "O1SL" {
          }
          frame "E2LB", "E2SC" {
          }
          frame "C1UL" {
          }
        }
        n205 = call "plc write string.vi"("error in"=w540, "value"="" ("Data"), "addr,tag"=w539) -> ("error out"=w533:errorcluster)  [unwired: 8 in]
        n206 = property class="Clust (严格)"(reference=w530, error in=w533) -> (reference out=w537:refnum<vi>, error out=w534:errorcluster, "Value"=w535:T48)
        n207 = Bundle By Name(cluster=w535, "PLC Info"="") -> (w536:T48)
        n208 = property class="Clust (严格)"(reference=w537, error in=w534, "Value"=w536) -> (error out=w532:errorcluster)  [unwired: 1 out]
      }
      frame "Init Test" {
        w554 = "" ("Scanner Data 1")
        w553 = FALSE
        n209 = Unbundle By Name(w552) -> ("SS Barcode Reader"=w564:refnum<visa-resource-name>, "SS barcode scanner ip"=w563:string, "hmi status indicator ref"=w551:refnum<vi>)
        n210 = Empty String/Path?(string/path=w563) -> (empty?=w562:bool)
        n211 = case shown="真" w562 {
          tunnel: w564 -> [_ w568]
          tunnel: [_ w567] -> w556
          tunnel: w561 -> [_ w566]
          frame False {
          }
          frame True {
            n212 = VISA Flush I/O Buffer(VISA resource name=w568, error in (no error)=w566) -> (error out=w567:errorcluster)  [unwired: 1 in, 1 out]
          }
        }
        n213 = property class="Clust (严格)"(reference=w551, error in=w556) -> (reference out=w560:refnum<vi>, error out=w558:errorcluster, "Value"=w559:T48)
        n214 = Bundle By Name(cluster=w559, "Scanner Data 1"=w554, "Scanner Data 2"=w554, "Serial Number"=w554, "Inalfa Part Number"=w554, "Color"=w554, "PLC Barcode Data 1"=w554, "PLC Barcode Data 2"=w554, "Model Type"=w554, "PHN"=w554, "Customer Number"=w554, "Scanner Data 1 Ok"=w553, "Scanner Data 2 Ok"=w553) -> (w557:T48)
        n215 = property class="Clust (严格)"(reference=w560, error in=w558, "Value"=w557) -> (error out=w555:errorcluster)  [unwired: 1 out]
      }
    }
    n216 = Unbundle By Name(w32) -> ("hmi status indicator ref"=w34:refnum<vi>)
    n217 = property class="Clust (严格)"(reference=w34) -> (reference out=w38:refnum<vi>, error out=w36:errorcluster, "Value"=w37:T48)  [unwired: 1 in]
    n218 = Bundle By Name(cluster=w37, "Station Application Status"=w33) -> (w35:T48)
    n219 = property class="Clust (严格)"(reference=w38, error in=w36, "Value"=w35) -> ()  [unwired: 2 out]
  }
  "error out" <- w1
